vi "Main.vi"() -> ()   [LabVIEW 2020]
uses:
  Control 2.ctl
  score.ctl
  <userlib>/_NEVSTOP/Communicable State Machine(CSM)/_Support/Priority Queue/Priority Queue.lvclass/Priority Queue.ctl
  c319eba2-2b69-4508-ba06-61efdf669e7f.vi
  f21c7960-0f7f-4192-a8ac-ee65138fb98e.vi
  0e5201a1-580a-4182-a838-348a54a2e186.vi
  50275f31-ecc9-42d7-9ef1-34fd3155a618.vi
  0e7b1505-b89c-402a-9fd1-9f3cfcf1be26.vi
  d7687cdb-357b-4687-95b9-9b4cfc2d17b9.vi
  52e50a07-fba7-4300-b081-eb3bf9999503.vi
  91789a72-074d-44cf-8be7-f4eccb61965a.vi
  5ff8236f-55fa-4ae3-afc0-cb7bd4a41e4f.vi
  <userlib>/_NEVSTOP/Communicable State Machine(CSM)/_Polymophic/Build No-Reply Asynchronous Message with Arguments.vi
  939ea49c-9fb9-49f6-a0c7-57a14fefe734.vi
  03371d6b-8044-40a1-9300-825b312c4f02.vi
  d32dd9c0-23c6-42c4-b7b9-cda287316cd3.vi
  d337f771-a6ec-4da6-9b1c-67b8dc694886.vi
  9b28357d-31d9-4419-b7a1-8921e76f82ac.vi
  67dfaec1-d8c9-4a60-939d-f2d06e17c127.vi
  ca159b87-ec92-4442-a782-4ab02e472262.vi
  a8ebcde1-3a60-408d-b02a-9696afebc65b.vi
  9c19e163-6e76-42e7-8cae-1a7d439f1586.vi
  <userlib>/_NEVSTOP/Communicable State Machine(CSM)/_Support/Process/CSMP-Async Call.vi
  <userlib>/_NEVSTOP/Communicable State Machine(CSM)/_Support/GlobalEvent/GEvt-Generate Status Log.vi
  <userlib>/_NEVSTOP/Communicable State Machine(CSM)/_Support/Process/CSMP-Broadcast.vi
  <userlib>/_NEVSTOP/Communicable State Machine(CSM)/_Support/GlobalEvent/GEvt-Generate Interrupt Log.vi
  <userlib>/_NEVSTOP/Communicable State Machine(CSM)/_Support/GlobalEvent/GEvt-Generate Register Log.vi
  <userlib>/_NEVSTOP/Communicable State Machine(CSM)/_Support/Process/CSMP-Register Status.vi
  <userlib>/_NEVSTOP/Communicable State Machine(CSM)/_Support/GlobalEvent/GEvt-Generate Unregister Log.vi
  <userlib>/_NEVSTOP/Communicable State Machine(CSM)/_Support/Process/CSMP-Unregister Status.vi
  <userlib>/_NEVSTOP/Communicable State Machine(CSM)/_Support/Process/CSMP-Sync Call.vi
  <userlib>/_NEVSTOP/Communicable State Machine(CSM)/_Support/CSMQ/_CSMObj-Unlock.vi
  <userlib>/_NEVSTOP/Communicable State Machine(CSM)/_Support/Process/CSMP-PostPostMsg.vi
  <userlib>/_NEVSTOP/Communicable State Machine(CSM)/_Support/Process/CSMP-PostSendMsg.vi
  <userlib>/_NEVSTOP/Communicable State Machine(CSM)/_Support/CSMQ/_CSMObj-Lock State.vi
  <userlib>/_NEVSTOP/Communicable State Machine(CSM)/_Support/Common/Splite Reason String Part.vi
  <userlib>/_NEVSTOP/Communicable State Machine(CSM)/_Support/Common/Trim Single line Text.vi
  <userlib>/_NEVSTOP/Communicable State Machine(CSM)/_Support/CSMQ/_CSMOFGV Release.vi
  <userlib>/_NEVSTOP/Communicable State Machine(CSM)/_Support/Common/Remove Comments from Line.vi
  <userlib>/_NEVSTOP/Communicable State Machine(CSM)/_Support/Common/Splite Single-line Message.vi
  <userlib>/_NEVSTOP/Communicable State Machine(CSM)/_Support/Common/Parse Next Single-line State.vi
  <userlib>/_NEVSTOP/Communicable State Machine(CSM)/_Support/CSMQ/_CSMOFGV Dequeue.vi
  <userlib>/_NEVSTOP/Communicable State Machine(CSM)/_Support/CSMQ/_CSMObj-Log Error if in a Remote Session.vi
  <userlib>/_NEVSTOP/Communicable State Machine(CSM)/_Support/GlobalEvent/GEvt-Generate State Change Log.vi
  <userlib>/_NEVSTOP/Communicable State Machine(CSM)/_Support/GlobalEvent/GEvt-Generate Remaining States Log.vi
  <userlib>/_NEVSTOP/Communicable State Machine(CSM)/_Support/GlobalEvent/GEvt-Generate Module Destroyed Log.vi
  <userlib>/_NEVSTOP/Communicable State Machine(CSM)/_Support/GlobalEvent/GEvt-Generate Complete Log.vi
  <userlib>/_NEVSTOP/Communicable State Machine(CSM)/_Support/GlobalEvent/GEvt-Generate Module Created Log.vi
  <userlib>/_NEVSTOP/Communicable State Machine(CSM)/_Support/GlobalEvent/Cache-GEvt Filter Object.vi
  <userlib>/_NEVSTOP/Communicable State Machine(CSM)/_Support/Common/Format Timestamp.vi
  <userlib>/_NEVSTOP/Communicable State Machine(CSM)/AdvanceAPI/CSM - Wait for Module to Be Alive.vi
  <userlib>/_NEVSTOP/Communicable State Machine(CSM)/AdvanceAPI/CSM - Send Message and Wait for Reply.vi
  <userlib>/_NEVSTOP/Communicable State Machine(CSM)/AdvanceAPI/CSM - Break Down Multiple States String.vi
  <userlib>/_NEVSTOP/Communicable State Machine(CSM)/AdvanceAPI/CSM - Compact Multiple States.vi
  <userlib>/_NEVSTOP/Communicable State Machine(CSM)/Utility/uuid.vi
  <userlib>/_NEVSTOP/Communicable State Machine(CSM)/Utility/Build Error Cluster.vi
  <userlib>/_NEVSTOP/Communicable State Machine(CSM)/Utility/Trim Both Whitespace.vi
  <userlib>/_NEVSTOP/Communicable State Machine(CSM)/AdvanceAPI/CSM - Revert Arguments-Safe String.vi
  <userlib>/_NEVSTOP/Communicable State Machine(CSM)/AdvanceAPI/CSM - Make String Arguments Safe.vi
  <userlib>/_NEVSTOP/Communicable State Machine(CSM)/_Support/CSMQ/_CSMObj-Message Check.vi
  <userlib>/_NEVSTOP/Communicable State Machine(CSM)/_Support/CSMQ/_CSMObj-Enqueue Cross-Module Message.vi
  <userlib>/_NEVSTOP/Communicable State Machine(CSM)/_Support/CSMQ/_CSMOFGV Get.vi
  <userlib>/_NEVSTOP/Communicable State Machine(CSM)/_Support/GlobalEvent/GEvt-Generate with Rule Check.vi
  <userlib>/_NEVSTOP/Communicable State Machine(CSM)/_Support/FGV-BroadcastRegistry/Cache-Broadcast Registry Search Result.vi
  <userlib>/_NEVSTOP/Communicable State Machine(CSM)/AdvanceAPI/CSM - Register Status Change.vi
  <userlib>/_NEVSTOP/Communicable State Machine(CSM)/AdvanceAPI/CSM - Unregister Status Change.vi
  <userlib>/_NEVSTOP/Communicable State Machine(CSM)/_Support/Common/Hex Str to U8 Data.vi
  <userlib>/_NEVSTOP/Communicable State Machine(CSM)/_Support/Common/Concatenate State with Arguments.vi
  <userlib>/_NEVSTOP/Communicable State Machine(CSM)/_Support/Common/U8 Data to Hex Str.vi
  <userlib>/_NEVSTOP/Communicable State Machine(CSM)/_Support/Priority Queue/Dequeue Element.vi
  <userlib>/_NEVSTOP/Communicable State Machine(CSM)/AdvanceAPI/CSM - Check If Module Exists.vi
  <userlib>/_NEVSTOP/Communicable State Machine(CSM)/AdvanceAPI/CSM - Keywords.vi
  <userlib>/_NEVSTOP/Communicable State Machine(CSM)/_Support/Priority Queue/Enqueue Element.vi
  <userlib>/_NEVSTOP/Communicable State Machine(CSM)/_Support/GlobalEvent/LogFilter/Filter Check.vi
  <userlib>/_NEVSTOP/Communicable State Machine(CSM)/_Support/CSMQ/_Obtain CSM Data Queue.vi
  <userlib>/_NEVSTOP/Communicable State Machine(CSM)/_Support/Priority Queue/Release Priority Queue.vi
  <userlib>/_NEVSTOP/Communicable State Machine(CSM)/_Support/Priority Queue/Obtain Priority Queue.vi
  <userlib>/_NEVSTOP/Communicable State Machine(CSM)/_Support/GlobalEvent/FGV-GlobalEventRef.vi
  <userlib>/_NEVSTOP/Communicable State Machine(CSM)/_Support/GlobalEvent/global-GEvnt Filter Change Flag.vi
  <userlib>/_NEVSTOP/Communicable State Machine(CSM)/FGV-GEvt Filter Obj.vi
  <userlib>/_NEVSTOP/Communicable State Machine(CSM)/_Support/CSMQ/_CSMOFGV Obtain.vi
  <userlib>/_NEVSTOP/Communicable State Machine(CSM)/_Support/GlobalEvent/LogFilter/CheckVIs/Group Check - CSM.vi
  <userlib>/_NEVSTOP/Communicable State Machine(CSM)/_Support/GlobalEvent/LogFilter/CheckVIs/Group Check - LogType.vi
  <userlib>/_NEVSTOP/Communicable State Machine(CSM)/_Support/GlobalEvent/LogFilter/CheckVIs/Group Check - State.vi
  <userlib>/_NEVSTOP/Communicable State Machine(CSM)/_Support/GlobalEvent/LogFilter/CheckVIs/CSM Check - LogType.vi
  <userlib>/_NEVSTOP/Communicable State Machine(CSM)/_Support/GlobalEvent/LogFilter/CheckVIs/CSM Check - State.vi
  <userlib>/_NEVSTOP/Communicable State Machine(CSM)/_Support/GlobalEvent/LogFilter/CheckVIs/CSM Check - StateType.vi
  <userlib>/_NEVSTOP/Communicable State Machine(CSM)/_Support/GlobalEvent/LogFilter/CheckVIs/Group Check - StateType.vi
  <userlib>/_NEVSTOP/Communicable State Machine(CSM)/_Support/CSMQ/_CSMOFGV.vi
  <userlib>/_NEVSTOP/Communicable State Machine(CSM)/_Support/Error/CSM Not Allowed Message.vi
  <userlib>/_NEVSTOP/Communicable State Machine(CSM)/_Support/GlobalEvent/FGV-StatusChangeEventRef.vi
  <userlib>/_NEVSTOP/Communicable State Machine(CSM)/_Support/FGV-BroadcastRegistry/global-CSMQ FGV Change Flag.vi
  <userlib>/_NEVSTOP/Communicable State Machine(CSM)/_Support/FGV-BroadcastRegistry/global-Broadcast Cache Change Flag.vi
  <userlib>/_NEVSTOP/Communicable State Machine(CSM)/_Support/BroadcastRegistry/HelperVI/Broadcast Item Key.vi
  <userlib>/_NEVSTOP/Communicable State Machine(CSM)/_Support/FGV-BroadcastRegistry/FGV-BroadcastRegistry.vi
  <userlib>/_NEVSTOP/Communicable State Machine(CSM)/_Support/Message/Parse Register Message.vi
  <userlib>/_NEVSTOP/Communicable State Machine(CSM)/_Support/Message/Parse Unregister Message.vi
  <userlib>/_NEVSTOP/Communicable State Machine(CSM)/addons/API-String-Arugments-Support/_Support/Data To API String Arguments.vi
  <userlib>/_NEVSTOP/Communicable State Machine(CSM)/_Support/Error/CSM No Target Error.vi
  <userlib>/_NEVSTOP/Communicable State Machine(CSM)/addons/API-String-Arugments-Support/_Support/Convert API String Arguments to Data(variant).vi
  <userlib>/_NEVSTOP/Communicable State Machine(CSM)/_Support/Message/Parse State with Arguments String.vi
  <userlib>/_NEVSTOP/Communicable State Machine(CSM)/_Support/Priority Queue/Priority Queue.lvclass
  <userlib>/_NEVSTOP/Communicable State Machine(CSM)/Communicable State Machine.lvlib
panel:
  out "time":dbl
  in  "Stop":bool
  out "State History":string="\r"
  in  "Name(\"\" to use uuid)":string="Main"
  in  "Init State(\"Macro: Initialize\")":string="Macro: Initialize"
  in  "Tab Control":T1
  in  "exit":bool
  in  "register":bool
  in  "log":bool
  in  "username":string
  in  "password":string
  in  "level":enum16{"simple", "medium", "hard"}(ring)
  in  "newgame":bool
  in  "logout":bool
  in  "ranking":bool
  in  "continue":bool
  in  "Boolean 4":bool
  in  "Boolean 3":bool
  in  "Boolean 2":bool
  in  "Boolean1":bool
  in  "exit2":bool
  in  "start2":bool
  in  "save":bool
  in  "pause":bool
  out "Score":T2
  out "Countdown":dbl
  in  "update":bool
  in  "Top":i32=1 min=1 max=10 step=1
  out "Data":string[][](array[string])
  in  "exit3":bool
  # "Player"
  # "Score"
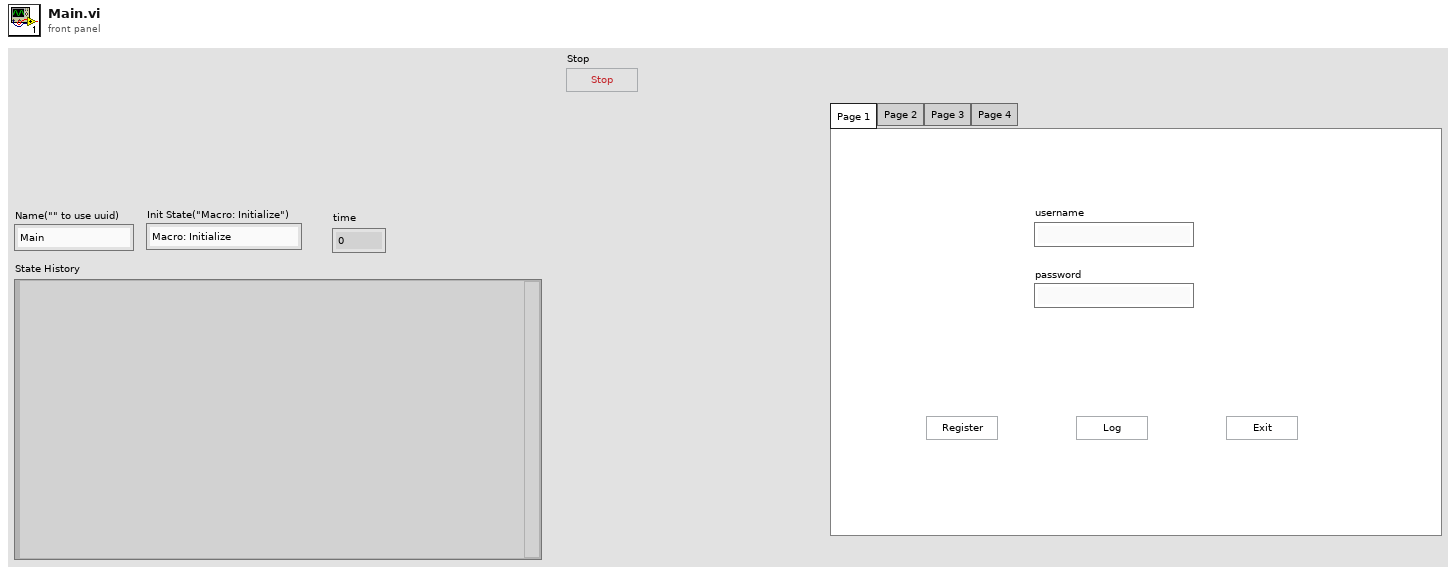
[diagram p1: front panel]
types:
  T1 = typedef "Control 2.ctl" = enum32{"Page 1", "Page 2", "Page 3", "Page 4"}
  T2 = typedef "score.ctl" = i32
  T3 = enum8{"Enabled", "Disabled", "Disabled and Grayed Out"}
  T4 = enum32{"Invalid", "Standard", "Closed", "Hidden", "Minimized", "Maximized"}
  T5 = enum32{"invalid app kind", "Development System", "Run Time System", "Student Edition", "Embedded LabVIEW", "Evaluation", "Custom"}
  T6 = typedef "Communicable State Machine.lvlib/_CSM_Response Source Message.ctl" = cluster{"‘State":string, "’Arguments":string, "’Error":errorcluster}
  T7 = cluster{"Tab Control":refnum<vi>, "start2":refnum<vi>, "Boolean1":refnum<vi>, "Boolean 3":refnum<vi>, "Boolean 4":refnum<vi>, "Boolean 2":refnum<vi>, "Core":cluster{"Current VI Reference":refnum<vi>, "Close Panel on Exit?":bool}, "rank":string[][], "ID":cluster{"username":string, "password":string}, "score":i32, "timeseq":cluster{"time":i32, "SEQ":i32[]}, "appended path":path, "start time":dbl, "Countdown":refnum<vi>}
  T8 = cluster{"Current VI Reference":refnum<vi>, "Close Panel on Exit?":bool}
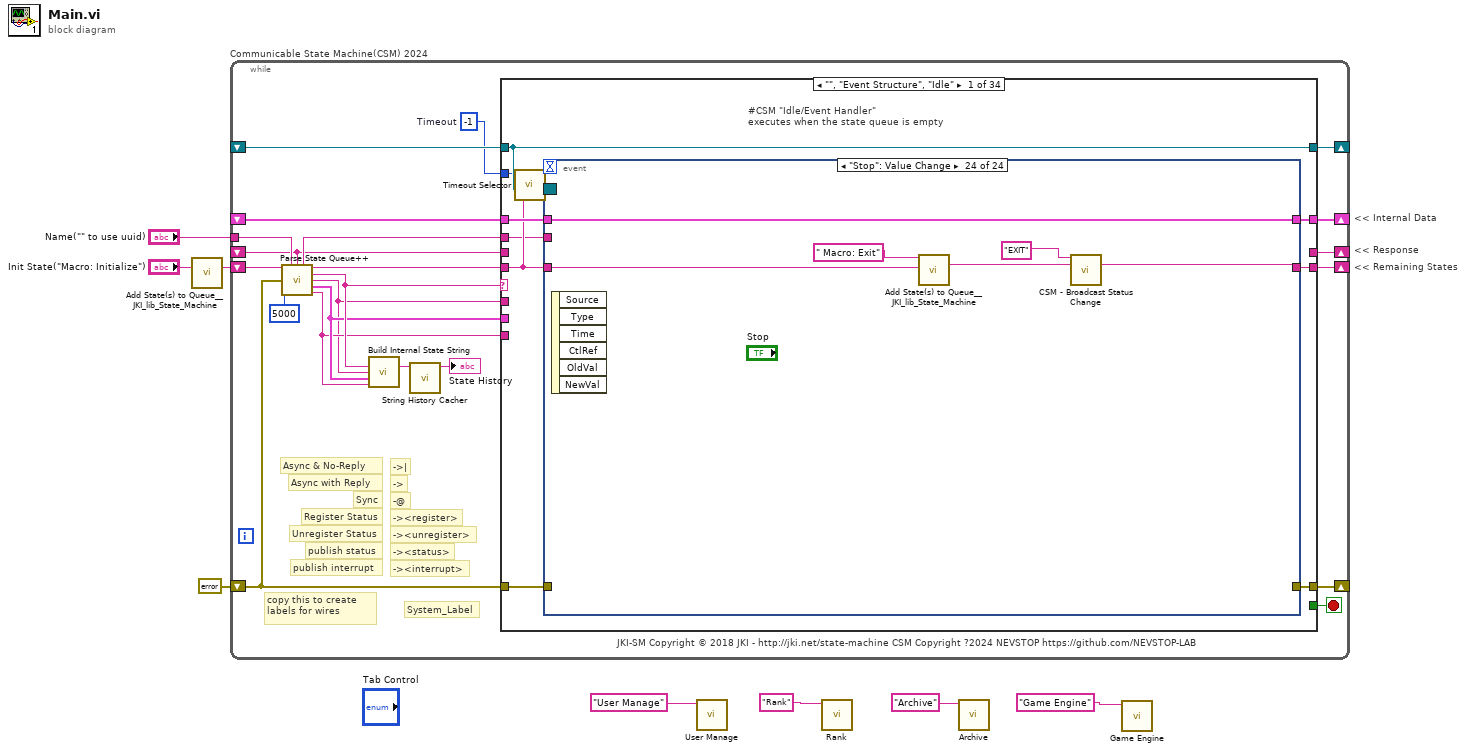
[diagram p0: block diagram]
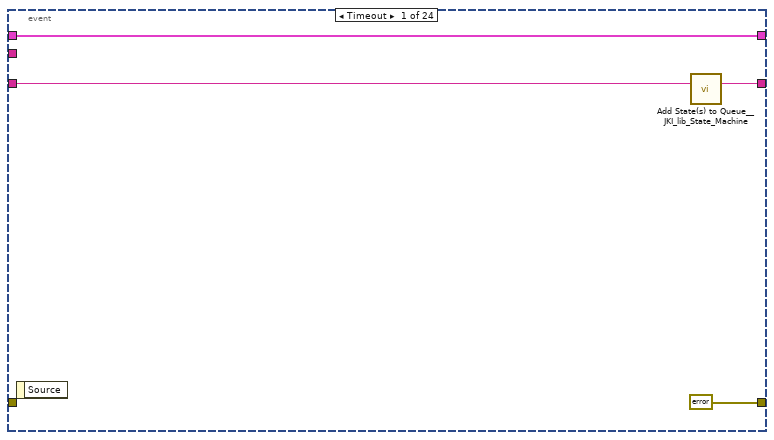
[diagram p2: hidden frame]
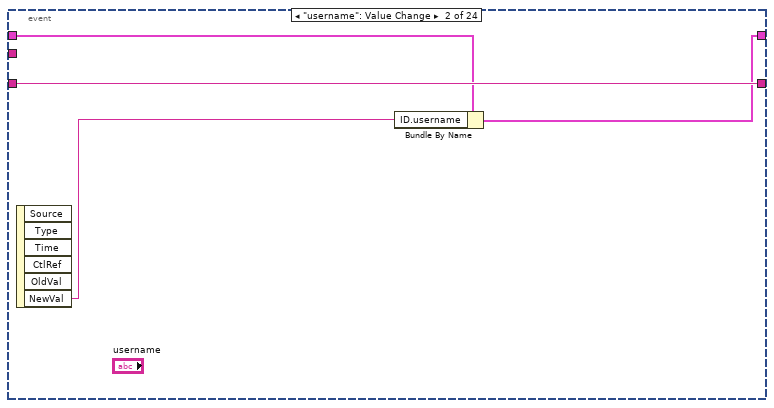
[diagram p3: hidden frame]
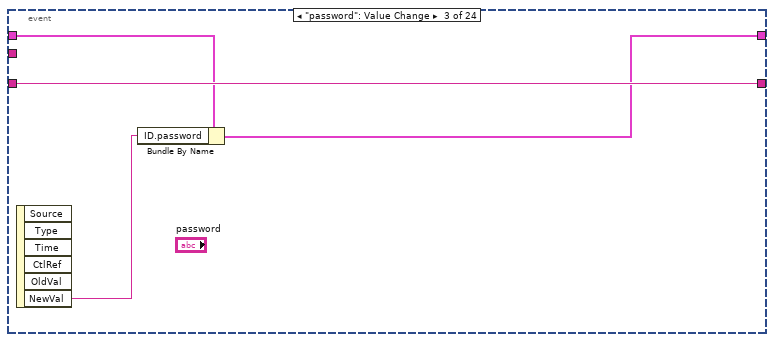
[diagram p4: hidden frame]
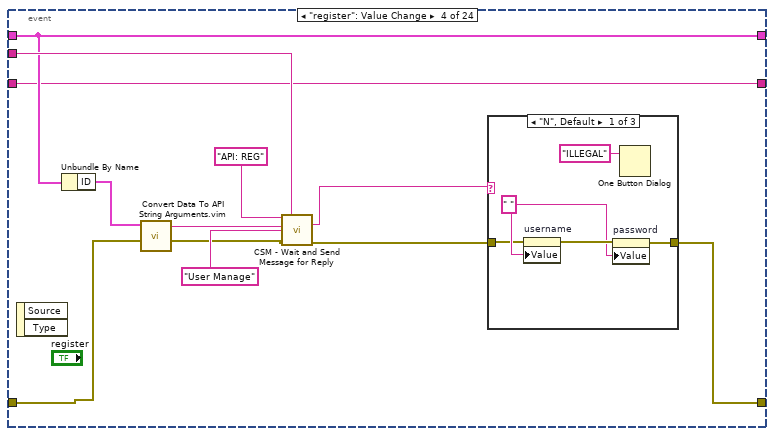
[diagram p5: hidden frame]
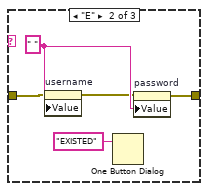
[diagram p6: hidden frame]
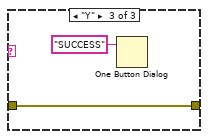
[diagram p7: hidden frame]
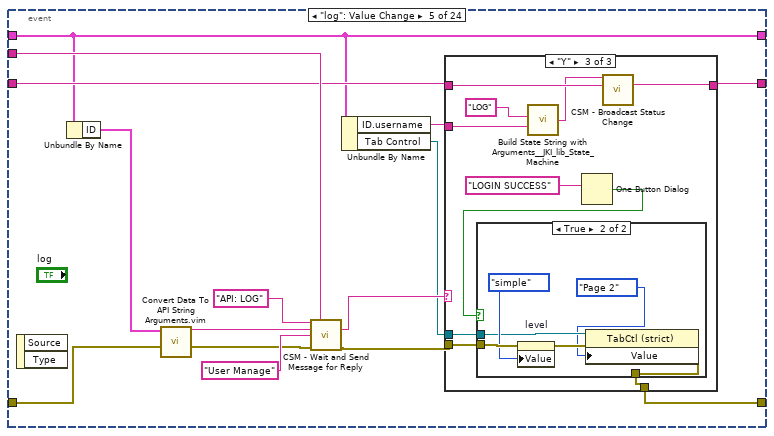
[diagram p8: hidden frame]
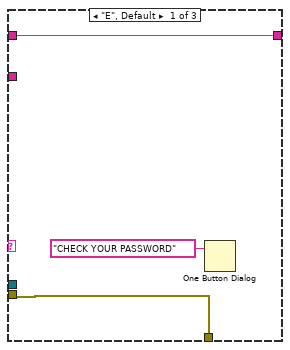
[diagram p9: hidden frame]
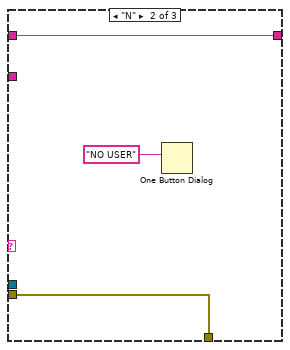
[diagram p10: hidden frame]
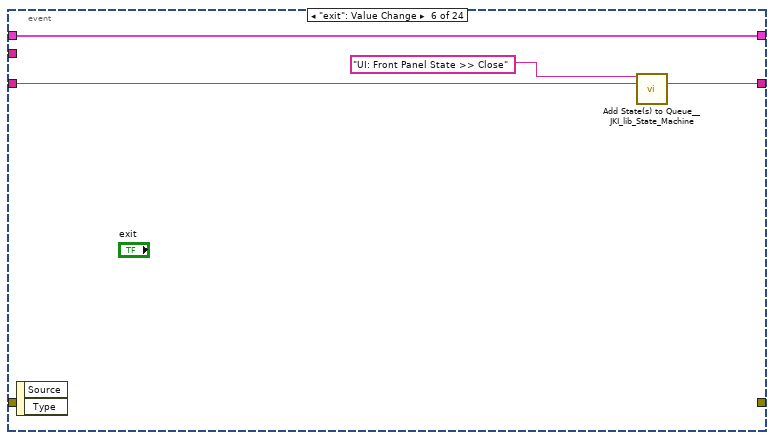
[diagram p12: hidden frame]
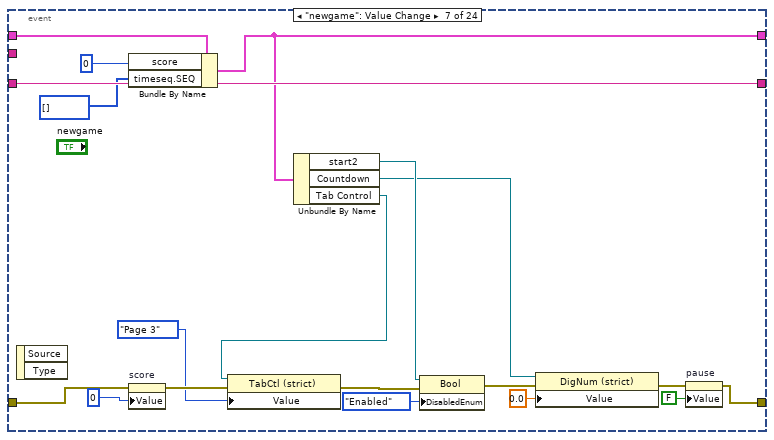
[diagram p13: hidden frame]
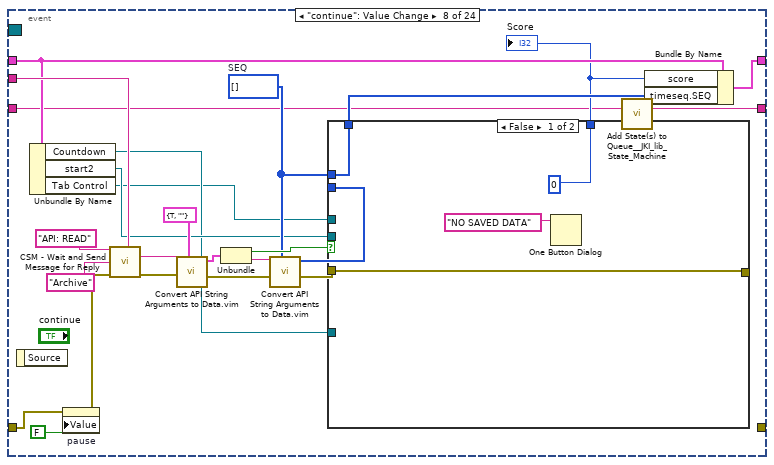
[diagram p14: hidden frame]
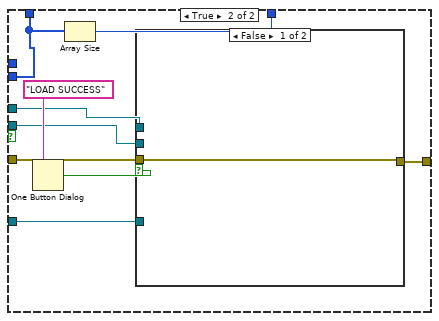
[diagram p15: hidden frame]
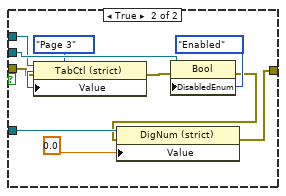
[diagram p16: hidden frame]
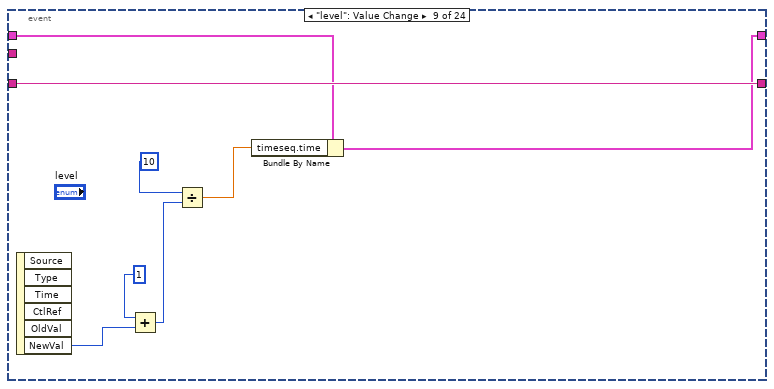
[diagram p17: hidden frame]
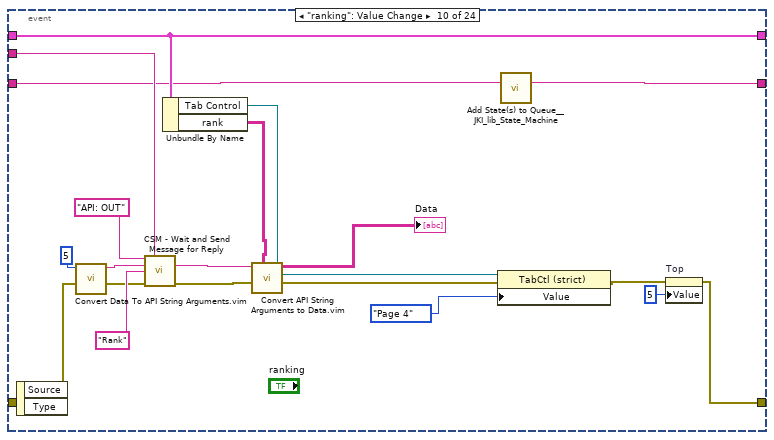
[diagram p18: hidden frame]
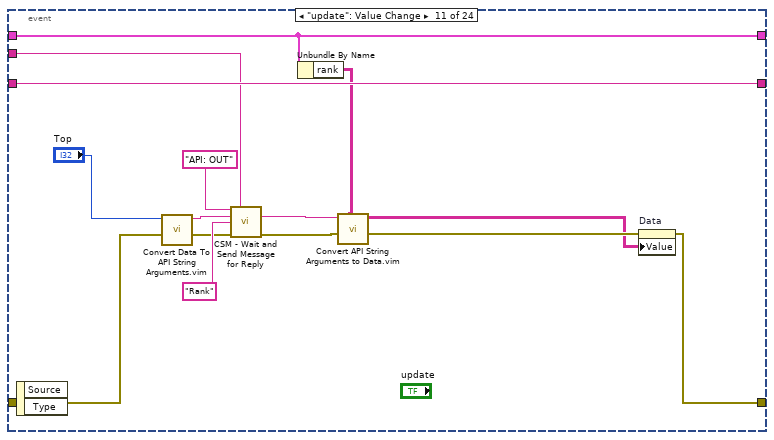
[diagram p19: hidden frame]
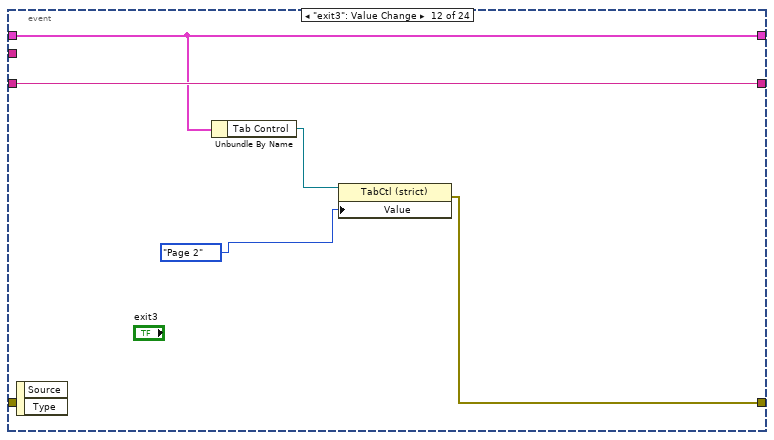
[diagram p20: hidden frame]
diagram:
  # "<< Internal Data"
  # "<< Response"
  # "<< Remaining States"
  n1 = call <vilib>:"Add State(s) to Queue__JKI_lib_State_Machine.vi"("State(s) in (\"\")"="Init State(\"Macro: Initialize\")") -> ("States Out"=w5:string)  [unwired: 14 in]
  n2 = while "Communicable State Machine(CSM) 2024" {
    shift-right: [w25] -> _
    shift-left: _ -> [w24]
    shift-right: [w28] -> _
    shift-left: errorcluster {"status"=FALSE, "code"=0, "source"=""} ("error out") -> [w23]
    shift-right: [w27] -> _
    shift-left: w5 -> [w29]
    tunnel: "Name(\"\" to use uuid)" -> [w18]
    shift-right: [w21] -> _
    shift-left: _ -> [w11]
    shift-right: [w20] -> _
    shift-left: _ -> [w19]
    stop <- w26 stop-if-true
    w9 = -1  # Timeout
    # "-><interrupt>"
    # "-><status>"
    # "-><unregister>"
    # "-><register>"
    # "-@"
    # "->"
    # "->|"
    # "publish interrupt"
    # "publish status"
    # "Unregister Status"
    # "Register Status"
    # "Sync"
    # "Async with Reply"
    # "Async & No-Reply"
    # "copy this to create labels for wires"
    # "System_Label"
    # "JKI-SM Copyright © 2018 JKI - http://jki.net/state-machine CSM Copyright ?2024 NEVSTOP https://github.com/NEVSTOP-LAB"
    n3 = call <userlib>:"Parse State Queue++.vi"("State Queue"=w29, "Name(\"\" to use uuid)"=w18, "Response Arguments"=w11, "Error In (no error)"=w23, "Response Timeout(5000ms)"=5000 ("Response Timeout(1000ms)")) -> ("Name Used"=w12:string, "Remaining States"=w30:string, "Current State"=w15:string, "Arguments"=w10:string, ">> Response Source Message >>"=w14:T6, ">> Source CSM >>"=w13:string)  [unwired: 5 in]
    n4 = call <userlib>:"Build Internal State String.vi"("State"=w15, "Arguments (\"\")"=w10, ">> Response Source Message >>"=w14, "Source (\"\")"=w13) -> ("State with Arguments"=w16:string)  [unwired: 11 in]
    n5 = call <userlib>:"String History Cacher.vi"("String"=w16) -> ("String Cache"=→"State History":string)  [unwired: 10 in]
    n6 = case shown="\"\", \"Event Structure\", \"Idle\"" w15 {
      selector: w15 -> [_ _ _ w405 _ _ _ _ _ _ _ _ _ _ _ _ _ _ _ _ _ _ _ _ _ _ _ _ _ _ _ _ _ _]
      tunnel: w30 -> [w34 w397 w402 w411 w417 w424 w451 w459 w466 w476 w485 w498 w503 w507 w527 w533 w537 w544 w548 w552 w577 w583 w596 w660 w665 w676 w679 w688 w731 w750 w770 w786 w801 w821]
      tunnel: w10 -> [_ _ _ _ _ w422 w447 w454 w462 w470 _ _ _ _ _ _ _ _ _ _ _ w579 w593 _ _ _ _ w692 w728 _ _ _ _ _]
      tunnel: w24 -> [w39 w396 w399 w409 w416 w430 w452 w457 w464 w474 w484 w492 w501 w505 _ w529 w535 w543 w547 w550 w574 w581 w594 w658 w663 w674 w678 w691 w724 w734 w777 w784 w798 w810]
      tunnel: [w38 _ w400 w403 w418 errorcluster {"status"=FALSE, "code"=0, "source"=""} ("error out") w444 w453 w460 w473 _ _ _ _ _ w530 _ w538 w546 _ w554 w580 w589 _ _ _ _ w684 w726 w739 w756 _ w794 w815] -> w28
      tunnel: w23 -> [w32 _ w400 w404 w418 w428 w445 w455 w461 _ _ _ _ _ _ _ _ _ _ _ w557 _ _ _ _ _ _ _ w727 w737 w762 _ w788 w802]
      tunnel: [w40 w397 w401 w410 w417 w426 w450 w458 w465 w477 w485 w497 w502 w506 w526 w532 w536 w544 w548 w551 w576 w582 w595 w659 w664 w675 w679 w689 w730 w751 w771 w785 w800 w820] -> w27
      tunnel: [_ _ _ _ _ _ TRUE _ _ _ _ _ TRUE _ _ _ _ _ _ _ _ _ _ _ _ _ _ _ _ _ _ _ _ _] -> w26
      tunnel: [w37 w396 w399 w409 w416 w430 w452 w457 w464 w475 w484 w496 w501 w505 w525 w529 w535 w543 w547 w550 w574 w581 w594 w658 w663 w674 w678 w686 w724 w733 w781 w784 w798 w810] -> w25
      tunnel: w13 -> [_ _ _ _ _ w421 _ _ _ w471 _ _ _ _ _ _ _ _ _ _ _ _ _ _ _ _ _ _ _ _ _ _ _ _]
      tunnel: w14 -> [_ _ _ _ _ w420 _ _ _ w472 _ _ _ _ _ _ _ _ _ _ _ _ _ _ _ _ _ _ _ _ _ _ _ _]
      tunnel: [_ _ _ "" w412 w419 _ _ _ _ _ _ _ _ _ _ _ _ _ _ _ _ _ _ _ _ _ _ _ _ _ _ _ _] -> w21
      tunnel: [w36 w395 w398 w407 w415 w429 w448 w456 w463 w478 w483 w486 w499 w504 w523 w528 w534 w542 w545 w549 w575 w578 w592 w657 w661 w667 w677 w694 w729 w752 w782 w783 w799 w819] -> w20
      tunnel: w19 -> [w36 w395 w398 w407 w415 w429 w448 w456 w463 w478 w483 w486 w499 w504 w523 w528 w534 _ w545 w549 w575 w578 w592 w657 w661 w667 w677 w694 w729 w752 w782 w783 w799 w819]
      tunnel: w12 -> [w33 _ _ w406 _ _ w446 _ _ _ _ _ _ _ _ _ _ w541 _ _ _ _ _ _ _ _ _ _ _ _ _ _ _ _]
      tunnel: w11 -> [_ _ _ _ _ w419 _ _ _ _ _ _ _ _ _ _ _ _ _ _ _ _ _ _ _ _ _ _ _ _ _ _ _ _]
      tunnel: w9 -> [w31 _ _ _ _ _ _ _ _ _ _ _ _ _ _ _ _ _ _ _ _ _ _ _ _ _ _ _ _ _ _ _ _ _]
      frame "", "Event Structure", "Idle" {
        # "#CSM \"Idle/Event Handler\"\nexecutes when the state queue is empty"
        n7 = call <userlib>:"Timeout Selector.vi"("Remaining States"=w34, "Timeout Expected"=w31) -> ("Timeout"=w35:i32)  [unwired: 5 in]
        n8 = event shown="[23] \"Stop\": Value Change" {
          selector: w36 -> [_ _ _ _ _ _ _ _ _ _ _ _ _ _ _ _ _ _ _ _ _ _ _ _]
          dyn-events: _ -> [_ _ _ _ _ _ _ _ _ _ _ _ _ _ _ _ _ _ _ _ _ _ _ _]
          timeout: w35 -> [_ _ _ _ _ _ _ _ _ _ _ _ _ _ _ _ _ _ _ _ _ _ _ _]
          tunnel: w34 -> [w44 w48 w52 w56 w82 w115 w137 w138 w194 w195 w229 w234 w246 w254 w266 w283 w329 w335 w347 w360 w373 w382 w388 w390]
          tunnel: [w43 w48 w52 w56 w83 w117 w137 w139 w194 w196 w229 w234 w246 w260 w267 w284 w328 w336 w348 w361 w374 w382 w387 w392] -> w40
          tunnel: w39 -> [w42 w47 w50 w62 w81 w118 w136 w159 w193 w205 w219 w233 w240 w259 w268 w291 w325 w333 w344 w358 w371 w383 w386 w394]
          tunnel: [errorcluster {"status"=FALSE, "code"=0, "source"=""} ("error out") _ _ w53 w84 _ w121 _ _ w202 w216 w230 w244 w249 w262 w280 w320 w331 w345 w356 w369 _ _ _] -> w38
          tunnel: [w42 w46 w49 w62 w81 w118 w132 w158 w188 w205 w219 w233 w241 w259 w268 w291 w325 w333 w344 w358 w371 w383 w386 w394] -> w37
          tunnel: w33 -> [_ _ _ w64 w85 _ _ w162 _ w213 w221 _ _ _ _ w281 _ _ _ _ _ _ _ _]
          tunnel: w32 -> [_ _ _ w58 w86 _ w135 w144 _ w207 w222 _ w237 w261 w263 w290 w322 _ _ _ _ _ _ _]
          event Timeout {
            n9 = event-data() -> ()  [unwired: 1 in, 1 out]
            n10 = call <vilib>:"Add State(s) to Queue__JKI_lib_State_Machine.vi"("State(s) in (\"\")"=w44) -> ("States Out"=w43:string)  [unwired: 14 in]
          }
          event "username": Value Change {
            n11 = event-data() -> ("NewVal"=w45:string)  [unwired: 1 in, 5 out]
            n12 = Bundle By Name(cluster=w47, "ID.username"=w45) -> (w46:T7)
          }
          event "password": Value Change {
            n13 = event-data() -> ("NewVal"=w51:string)  [unwired: 1 in, 5 out]
            n14 = Bundle By Name(cluster=w50, "ID.password"=w51) -> (w49:T7)
          }
          event "register": Value Change {
            n15 = event-data() -> ()  [unwired: 1 in, 2 out]
            n16 = Unbundle By Name(w62) -> ("ID"=w61:cluster{"username":string, "password":string})
            n17 = call "Convert Data To API String Arguments.vim"("error in (no error)"=w58, "data"=w61) -> ("error out"=w57:errorcluster, "String"=w60:string)  [unwired: 6 in]
            n18 = call <userlib>:"CSM - Wait and Send Message for Reply.vi"("State"="API: REG", "Current Module(\"\" to generate a ID)"=w64, "Arguments (\"\")"=w60, "Target Module"="User Manage", "Error In (no error)"=w57) -> ("Response"=w55:string, "error out"=w54:errorcluster)  [unwired: 8 in, 1 out]
            n19 = case shown="\"N\", Default" w55 {
              tunnel: w54 -> [w65 w72 w75]
              tunnel: [w66 w70 w75] -> w53
              frame "N", Default {
                w67 = " " ("username")
                n20 = property on="username" class="Str"(error in=w65, "Value"=w67) -> (error out=w68:errorcluster)  [unwired: 1 in, 1 out]
                n21 = property on="password" class="Str"(error in=w68, "Value"=w67) -> (error out=w66:errorcluster)  [unwired: 1 in, 1 out]
                n22 = One Button Dialog(message="ILLEGAL") -> ()  [unwired: 1 in, 1 out]
              }
              frame "E" {
                w73 = " " ("username")
                n23 = property on="username" class="Str"(error in=w72, "Value"=w73) -> (error out=w71:errorcluster)  [unwired: 1 in, 1 out]
                n24 = One Button Dialog(message="EXISTED") -> ()  [unwired: 1 in, 1 out]
                n25 = property on="password" class="Str"(error in=w71, "Value"=w73) -> (error out=w70:errorcluster)  [unwired: 1 in, 1 out]
              }
              frame "Y" {
                n26 = One Button Dialog(message="SUCCESS") -> ()  [unwired: 1 in, 1 out]
              }
            }
          }
          event "log": Value Change {
            n27 = event-data() -> ()  [unwired: 1 in, 2 out]
            n28 = Unbundle By Name(w81) -> ("ID"=w90:cluster{"username":string, "password":string})
            n29 = call "Convert Data To API String Arguments.vim"("error in (no error)"=w86, "data"=w90) -> ("error out"=w87:errorcluster, "String"=w89:string)  [unwired: 6 in]
            n30 = call <userlib>:"CSM - Wait and Send Message for Reply.vi"("State"="API: LOG", "Current Module(\"\" to generate a ID)"=w85, "Arguments (\"\")"=w89, "Target Module"="User Manage", "Error In (no error)"=w87) -> ("Response"=w78:string, "error out"=w79:errorcluster)  [unwired: 8 in, 1 out]
            n31 = Unbundle By Name(w81) -> ("ID.username"=w80:string, "Tab Control"=w77:refnum<vi>)
            n32 = case shown="\"Y\"" w78 {
              tunnel: w79 -> [w93 w96 w105]
              tunnel: [w93 w96 w104] -> w84
              tunnel: [w92 w95 w102] -> w83
              tunnel: w82 -> [w92 w95 w103]
              tunnel: w80 -> [_ _ w100]
              tunnel: w77 -> [_ _ w98]
              frame "E", Default {
                n33 = One Button Dialog(message="CHECK YOUR PASSWORD") -> ()  [unwired: 1 in, 1 out]
              }
              frame "N" {
                n34 = One Button Dialog(message="NO USER") -> ()  [unwired: 1 in, 1 out]
              }
              frame "Y" {
                n35 = call <vilib>:"Build State String with Arguments__JKI_lib_State_Machine.vi"("Arguments (\"\")"=w100, "State"="LOG") -> ("State with Arguments"=w101:string)  [unwired: 4 in]
                n36 = One Button Dialog(message="LOGIN SUCCESS") -> (true=w106:bool)  [unwired: 1 in]
                n37 = case shown="True" w106 {
                  tunnel: w105 -> [w108 w114]
                  tunnel: [w108 w110] -> w104
                  tunnel: w98 -> [_ w111]
                  frame False {
                  }
                  frame True {
                    n38 = property on="level" class="Enum (strict)"(error in=w114, "Value"=enum16{"simple", "medium", "hard"}."simple" ("level")) -> (error out=w112:errorcluster)  [unwired: 1 in, 1 out]
                    n39 = property class="TabCtl (strict)"(reference=w111, error in=w112, "Value"=Control_2."Page 2" ("Tab Control")) -> (error out=w110:errorcluster)  [unwired: 1 out]
                  }
                }
                n40 = call <userlib>:"CSM - Broadcast Status Change.vi"("Status with Arguments"=w101, "State Queue"=w103) -> ("Remaining States"=w102:string)  [unwired: 13 in]
              }
            }
          }
          event "exit": Value Change {
            n41 = event-data() -> ()  [unwired: 1 in, 2 out]
            n42 = call <vilib>:"Add State(s) to Queue__JKI_lib_State_Machine.vi"("State(s) in Front (\"\")"="UI: Front Panel State >> Close" ("State(s) in Front (\"\")"), "State(s) in (\"\")"=w115) -> ("States Out"=w117:string)  [unwired: 13 in]
          }
          event "newgame": Value Change {
            n43 = event-data() -> ()  [unwired: 1 in, 2 out]
            n44 = Bundle By Name(cluster=w136, "score"=0, "timeseq.SEQ"=i32[] [] ("SEQ")) -> (w132:T7)
            n45 = property on="score" class="DigNum (strict)"(error in=w135, "Value"=T2 0 ("score")) -> (error out=w126:errorcluster)  [unwired: 1 in, 1 out]
            n46 = Unbundle By Name(w132) -> ("start2"=w131:refnum<vi>, "Countdown"=w129:refnum<vi>, "Tab Control"=w123:refnum<vi>)
            n47 = property class="TabCtl (strict)"(reference=w123, error in=w126, "Value"=Control_2."Page 3" ("Tab Control")) -> (error out=w125:errorcluster)  [unwired: 1 out]
            n48 = property class="Bool"(reference=w131, error in=w125, "DisabledEnum"=T3."Enabled" ("Disabled")) -> (error out=w128:errorcluster)  [unwired: 1 out]
            n49 = property class="DigNum (strict)"(reference=w129, error in=w128, "Value"=0.0) -> (error out=w122:errorcluster)  [unwired: 1 out]
            n50 = property on="pause" class="Bool (strict)"(error in=w122, "Value"=FALSE ("pause")) -> (error out=w121:errorcluster)  [unwired: 1 in, 1 out]
          }
          event "continue": Value Change {
            w147 = i32[] []  # SEQ
            n51 = event-data() -> ()  [unwired: 1 in, 1 out]
            n52 = Unbundle By Name(w159) -> ("Countdown"=w141:refnum<vi>, "start2"=w142:refnum<vi>, "Tab Control"=w140:refnum<vi>)
            n53 = property on="pause" class="Bool (strict)"(error in=w144, "Value"=FALSE ("pause")) -> (error out=w143:errorcluster)  [unwired: 1 in, 1 out]
            n54 = call <userlib>:"CSM - Wait and Send Message for Reply.vi"("State"="API: READ", "Current Module(\"\" to generate a ID)"=w162, "Target Module"="Archive", "Error In (no error)"=w143) -> ("Response"=w156:string, "error out"=w157:errorcluster)  [unwired: 9 in, 1 out]
            n55 = call "Convert API String Arguments to Data.vim"("Type"=cluster{"found?":bool, "value":string} {"found?"=TRUE, "value"=""}, "error in (no error)"=w157, "String"=w156) -> ("error"=w150:errorcluster, "Data"=w154:cluster{"found?":bool, "value":string})  [unwired: 5 in]
            n56 = Unbundle(w154) -> ("found?"=w153:bool, "value"=w152:string)
            n57 = call "Convert API String Arguments to Data.vim"("Type"=w147, "error in (no error)"=w150, "String"=w152) -> ("error"=w149:errorcluster, "Data"=w151:i32[])  [unwired: 5 in]
            n58 = case shown="False" w153 {
              tunnel: w149 -> [w164 w173]
              tunnel: [0 ("score") w171] -> w146
              tunnel: [w164 w172] -> _
              tunnel: w151 -> [_ w170]
              tunnel: [w163 w170] -> w148
              tunnel: w147 -> [w163 _]
              tunnel: w142 -> [_ w169]
              tunnel: w141 -> [_ w168]
              tunnel: w140 -> [_ w167]
              frame False {
                n59 = One Button Dialog(message="NO SAVED DATA") -> ()  [unwired: 1 in, 1 out]
              }
              frame True {
                n60 = One Button Dialog(message="LOAD SUCCESS") -> (true=w174:bool)  [unwired: 1 in]
                n61 = Array Size(array=w170) -> (size(s)=w171:i32)
                n62 = case shown="False" w174 {
                  tunnel: w173 -> [w176 w178]
                  tunnel: [w176 w181] -> w172
                  tunnel: w169 -> [_ w184]
                  tunnel: w168 -> [_ w183]
                  tunnel: w167 -> [_ w177]
                  frame False {
                  }
                  frame True {
                    n63 = property class="TabCtl (strict)"(reference=w177, error in=w178, "Value"=Control_2."Page 3" ("Tab Control")) -> (error out=w179:errorcluster)  [unwired: 1 out]
                    n64 = property class="Bool"(reference=w184, error in=w179, "DisabledEnum"=T3."Enabled" ("Disabled")) -> (error out=w182:errorcluster)  [unwired: 1 out]
                    n65 = property class="DigNum (strict)"(reference=w183, error in=w182, "Value"=0.0) -> (error out=w181:errorcluster)  [unwired: 1 out]
                  }
                }
              }
            }
            "Score" <- w146
            n66 = call <vilib>:"Add State(s) to Queue__JKI_lib_State_Machine.vi"("State(s) in (\"\")"=w138) -> ("States Out"=w139:string)  [unwired: 14 in]
            n67 = Bundle By Name(cluster=w159, "score"=w146, "timeseq.SEQ"=w148) -> (w158:T7)
          }
          event "level": Value Change {
            n68 = event-data() -> ("NewVal"=w192:enum16{"simple", "medium", "hard"})  [unwired: 1 in, 5 out]
            n69 = Add(x=1, y=w192) -> (x+y=w190:i32)
            n70 = Divide(x=10, y=w190) -> (x/y=w187:dbl)
            n71 = Bundle By Name(cluster=w193, "timeseq.time"=w187) -> (w188:T7)
          }
          event "ranking": Value Change {
            n72 = event-data() -> ()  [unwired: 1 in, 2 out]
            n73 = call "Convert Data To API String Arguments.vim"("error in (no error)"=w207, "data"=5 ("top")) -> ("error out"=w208:errorcluster, "String"=w209:string)  [unwired: 6 in]
            n74 = call <userlib>:"CSM - Wait and Send Message for Reply.vi"("State"="API: OUT", "Current Module(\"\" to generate a ID)"=w213, "Arguments (\"\")"=w209, "Target Module"="Rank", "Error In (no error)"=w208) -> ("Response"=w211:string, "error out"=w210:errorcluster)  [unwired: 8 in, 1 out]
            n75 = Unbundle By Name(w205) -> ("Tab Control"=w197:refnum<vi>, "rank"=w204:string[][])
            n76 = call "Convert API String Arguments to Data.vim"("Type"=w204, "error in (no error)"=w210, "String"=w211) -> ("error"=w200:errorcluster, "Data"=→"Data":string[][])  [unwired: 5 in]
            n77 = property class="TabCtl (strict)"(reference=w197, error in=w200, "Value"=Control_2."Page 4" ("Tab Control")) -> (error out=w199:errorcluster)  [unwired: 1 out]
            n78 = call <vilib>:"Add State(s) to Queue__JKI_lib_State_Machine.vi"("State(s) in (\"\")"=w195) -> ("States Out"=w196:string)  [unwired: 14 in]
            n79 = property on="Top" class="DigNum (strict)"(error in=w199, "Value"=5 ("top")) -> (error out=w202:errorcluster)  [unwired: 1 in, 1 out]
          }
          event "update": Value Change {
            n80 = event-data() -> ()  [unwired: 1 in, 2 out]
            n81 = call "Convert Data To API String Arguments.vim"("error in (no error)"=w222, "data"="Top") -> ("error out"=w223:errorcluster, "String"=w224:string)  [unwired: 6 in]
            n82 = call <userlib>:"CSM - Wait and Send Message for Reply.vi"("State"="API: OUT", "Current Module(\"\" to generate a ID)"=w221, "Arguments (\"\")"=w224, "Target Module"="Rank", "Error In (no error)"=w223) -> ("Response"=w226:string, "error out"=w225:errorcluster)  [unwired: 8 in, 1 out]
            n83 = Unbundle By Name(w219) -> ("rank"=w218:string[][])
            n84 = call "Convert API String Arguments to Data.vim"("Type"=w218, "error in (no error)"=w225, "String"=w226) -> ("error"=w217:errorcluster, "Data"=w215:string[][])  [unwired: 5 in]
            n85 = property on="Data" class="Arr (strict)"(error in=w217, "Value"=w215) -> (error out=w216:errorcluster)  [unwired: 1 in, 1 out]
          }
          event "exit3": Value Change {
            n86 = event-data() -> ()  [unwired: 1 in, 2 out]
            n87 = Unbundle By Name(w233) -> ("Tab Control"=w232:refnum<vi>)
            n88 = property class="TabCtl (strict)"(reference=w232, "Value"=Control_2."Page 2" ("Tab Control")) -> (error out=w230:errorcluster)  [unwired: 1 in, 1 out]
          }
          event "logout": Value Change {
            w242 = "" ("ID.username")
            w243 = "" ("password")
            n89 = event-data() -> ()  [unwired: 1 in, 2 out]
            n90 = Unbundle By Name(w240) -> ("Tab Control"=w239:refnum<vi>)
            n91 = Bundle By Name(cluster=w240, "ID.username"=w242, "ID.password"=w242, "timeseq.time"=10) -> (w241:T7)
            n92 = property class="TabCtl (strict)"(reference=w239, error in=w237, "Value"=Control_2."Page 1" ("Tab Control")) -> (error out=w236:errorcluster)  [unwired: 1 out]
            n93 = property on="password" class="Str"(error in=w236, "Value"=w243) -> (error out=w245:errorcluster)  [unwired: 1 in, 1 out]
            n94 = property on="username" class="Str"(error in=w245, "Value"=w243) -> (error out=w244:errorcluster)  [unwired: 1 in, 1 out]
          }
          event "start2": Value Change {
            n95 = event-data() -> ()  [unwired: 1 in, 4 out]
            n96 = Unbundle By Name(w259) -> ("timeseq"=w248:cluster{"time":i32, "SEQ":i32[]})
            n97 = call "Convert Data To API String Arguments.vim"("error in (no error)"=w261, "data"=w248) -> ("error out"=w250:errorcluster, "String"=w257:string)  [unwired: 6 in]
            n98 = call <vilib>:"Add State(s) to Queue__JKI_lib_State_Machine.vi"("State(s) in (\"\")"=w254) -> ("States Out"=w255:string)  [unwired: 14 in]
            n99 = call-poly <userlib>:"Build Message with Arguments++.vi"("State with Arguments"="API: SEQ" ("State"), "Arguments (\"\")"=w257, "Target Module (\"\")"="Game Engine" ("Target Module")) -> ("State with Arguments out"=w253:string)  [unwired: 12 in]
            n100 = call <vilib>:"Add State(s) to Queue__JKI_lib_State_Machine.vi"("State(s) in Front (\"\")"="Action: DISABLE" ("State(s) in Front (\"\")"), "State(s) in (\"\")"=w253) -> ("States Out"=w247:string)  [unwired: 13 in]
            n101 = property on="start2" class="Bool"(error in=w250, "DisabledEnum"=T3."Disabled and Grayed Out" ("Disabled")) -> (error out=w249:errorcluster)  [unwired: 1 in, 1 out]
            n102 = call <vilib>:"Add State(s) to Queue__JKI_lib_State_Machine.vi"("State(s) in Front (\"\")"=w247, "State(s) in (\"\")"=w255) -> ("States Out"=w260:string)  [unwired: 13 in]
          }
          event "pause": Value Change {
            n103 = event-data() -> ("NewVal"=w265:bool)  [unwired: 1 in, 5 out]
            n104 = case shown="False" w265 {
              tunnel: [w274 w277] -> w264
              tunnel: w263 -> [w270 w276]
              tunnel: [w269 w276] -> w262
              frame False {
                n105 = Get Date/Time In Seconds() -> (seconds since 1Jan1904=w272:timestamp)
                n106 = call "Convert Data To API String Arguments.vim"("error in (no error)"=w270, "data"=w272) -> ("error out"=w269:errorcluster, "String"=w271:string)  [unwired: 6 in]
                n107 = call-poly <userlib>:"Build Message with Arguments++.vi"("State with Arguments"="API: RESUME", "Arguments (\"\")"=w271, "Target Module (\"\")"="Game Engine" ("Target Module (\"\")")) -> ("State with Arguments out"=w274:string)  [unwired: 12 in]
              }
              frame True {
                n108 = call-poly <userlib>:"Build Message with Arguments++.vi"("State with Arguments"="API: PAUSE", "Target Module (\"\")"="Game Engine" ("Target Module (\"\")")) -> ("State with Arguments out"=w277:string)  [unwired: 13 in]
              }
            }
            n109 = call <vilib>:"Add State(s) to Queue__JKI_lib_State_Machine.vi"("State(s) in Front (\"\")"=w264, "State(s) in (\"\")"=w266) -> ("States Out"=w267:string)  [unwired: 13 in]
          }
          event "save": Value Change {
            n110 = event-data() -> ()  [unwired: 1 in, 4 out]
            n111 = Unbundle By Name(w291) -> ("timeseq.SEQ"=w285:i32[])
            n112 = call "Convert Data To API String Arguments.vim"("error in (no error)"=w290, "data"=w285) -> ("error out"=w288:errorcluster, "String"=w289:string)  [unwired: 6 in]
            n113 = call <userlib>:"CSM - Wait and Send Message for Reply.vi"("State"="API: SAVE", "Current Module(\"\" to generate a ID)"=w281, "Arguments (\"\")"=w289, "Target Module"="Archive", "Error In (no error)"=w288) -> ("Response"=w286:string, "error out"=w282:errorcluster)  [unwired: 8 in, 1 out]
            n114 = case shown="\"Y\", Default" w286 {
              tunnel: w282 -> [w293 w295]
              tunnel: w281 -> [_ w298]
              tunnel: [w293 w297] -> w280
              frame "False" {
              }
              frame "Y", Default {
                n115 = property on="pause" class="Bool (strict)"(error in=w295) -> (error out=w294:errorcluster, "Value"=w296:bool)  [unwired: 1 in, 1 out]
                n116 = case shown="True" w296 {
                  tunnel: w294 -> [w303 w316]
                  tunnel: w298 -> [w302 _]
                  tunnel: [w300 w316] -> w297
                  frame False {
                    n117 = One Button Dialog(message="SAVE SUCCESS") -> (true=w299:bool)  [unwired: 1 in]
                    n118 = call <userlib>:"CSM - Post Message.vi"("Current Module(\"\" to generate a ID)"=w302, "Error In (no error)"=w303, "Target Module"="Game Engine" ("Target Module (\"\")"), "State"="API: PAUSE" ("State with Arguments")) -> ("error out"=w301:errorcluster)  [unwired: 7 in]
                    n119 = case shown="False" w299 {
                      tunnel: w302 -> [_ w311]
                      tunnel: w301 -> [w307 w310]
                      tunnel: [w307 w308] -> w300
                      frame False {
                      }
                      frame True {
                        n120 = Get Date/Time In Seconds() -> (seconds since 1Jan1904=w315:timestamp)
                        n121 = call "Convert Data To API String Arguments.vim"("error in (no error)"=w310, "data"=w315) -> ("error out"=w309:errorcluster, "String"=w312:string)  [unwired: 6 in]
                        n122 = call <userlib>:"CSM - Post Message.vi"("Current Module(\"\" to generate a ID)"=w311, "Error In (no error)"=w309, "Target Module"="Game Engine" ("Target Module (\"\")"), "Arguments (\"\")"=w312, "State"="API: RESUME" ("State with Arguments")) -> ("error out"=w308:errorcluster)  [unwired: 6 in]
                      }
                    }
                  }
                  frame True {
                    n123 = One Button Dialog(message="SAVE SUCCESS") -> ()  [unwired: 1 in, 1 out]
                  }
                }
              }
            }
            n124 = call <vilib>:"Add State(s) to Queue__JKI_lib_State_Machine.vi"("State(s) in (\"\")"=w283) -> ("States Out"=w284:string)  [unwired: 14 in]
          }
          event "exit2": Value Change {
            n125 = event-data() -> ()  [unwired: 1 in, 4 out]
            n126 = Unbundle By Name(w325) -> ("score"=w324:i32, "Tab Control"=w318:refnum<vi>)
            n127 = call "Convert Data To API String Arguments.vim"("error in (no error)"=w322, "data"=w324) -> ("error out"=w321:errorcluster, "String"=w323:string)  [unwired: 6 in]
            n128 = call <vilib>:"Build State String with Arguments__JKI_lib_State_Machine.vi"("Arguments (\"\")"=w323, "State"="GAMEEXIT") -> ("State with Arguments"=w327:string)  [unwired: 4 in]
            n129 = property class="TabCtl (strict)"(reference=w318, error in=w321, "Value"=Control_2."Page 2" ("Tab Control")) -> (error out=w320:errorcluster)  [unwired: 1 out]
            n130 = call <userlib>:"CSM - Broadcast Status Change.vi"("Status with Arguments"=w327, "State Queue"=w329) -> ("Remaining States"=w328:string)  [unwired: 13 in]
          }
          event "Boolean1": Value Change {
            n131 = event-data() -> ()  [unwired: 1 in, 6 out]
            n132 = call-poly <userlib>:"Build Message with Arguments++.vi"("State with Arguments"="API: TAP" ("State"), "Arguments (\"\")"="1" ("Arguments (\"\")"), "Target Module (\"\")"="Game Engine" ("Target Module")) -> ("State with Arguments out"=w334:string)  [unwired: 12 in]
            n133 = flat-sequence {
              tunnel: w332 -> [w341]
              tunnel: [w340] -> w331
              frame #0 {
                n134 = Wait (ms)(milliseconds to wait=u32 100) -> ()  [unwired: 1 out]
              }
              frame #1 {
                n135 = property class="Bool (strict)"(reference=w341, "Value"=FALSE ("Boolean1")) -> (error out=w340:errorcluster)  [unwired: 1 in, 1 out]
              }
            }
            n136 = call <vilib>:"Add State(s) to Queue__JKI_lib_State_Machine.vi"("State(s) in Front (\"\")"=w334, "State(s) in (\"\")"=w335) -> ("States Out"=w336:string)  [unwired: 13 in]
            n137 = Unbundle By Name(w333) -> ("Boolean1"=w332:refnum<vi>)
          }
          event "Boolean 2": Value Change {
            n138 = event-data() -> ()  [unwired: 1 in, 6 out]
            n139 = call-poly <userlib>:"Build Message with Arguments++.vi"("State with Arguments"="API: TAP" ("State"), "Arguments (\"\")"="2" ("Arguments (\"\")"), "Target Module (\"\")"="Game Engine" ("Target Module")) -> ("State with Arguments out"=w346:string)  [unwired: 12 in]
            n140 = flat-sequence {
              tunnel: [w354] -> w345
              tunnel: w343 -> [w353]
              frame #0 {
                n141 = Wait (ms)(milliseconds to wait=u32 100) -> ()  [unwired: 1 out]
              }
              frame #1 {
                n142 = property class="Bool (strict)"(reference=w353, "Value"=FALSE ("Boolean 2")) -> (error out=w354:errorcluster)  [unwired: 1 in, 1 out]
              }
            }
            n143 = Unbundle By Name(w344) -> ("Boolean 2"=w343:refnum<vi>)
            n144 = call <vilib>:"Add State(s) to Queue__JKI_lib_State_Machine.vi"("State(s) in Front (\"\")"=w346, "State(s) in (\"\")"=w347) -> ("States Out"=w348:string)  [unwired: 13 in]
          }
          event "Boolean 3": Value Change {
            n145 = event-data() -> ()  [unwired: 1 in, 6 out]
            n146 = call-poly <userlib>:"Build Message with Arguments++.vi"("State with Arguments"="API: TAP" ("State"), "Arguments (\"\")"="3" ("Arguments (\"\")"), "Target Module (\"\")"="Game Engine" ("Target Module")) -> ("State with Arguments out"=w359:string)  [unwired: 12 in]
            n147 = flat-sequence {
              tunnel: w357 -> [w367]
              tunnel: [w366] -> w356
              frame #0 {
                n148 = Wait (ms)(milliseconds to wait=u32 100) -> ()  [unwired: 1 out]
              }
              frame #1 {
                n149 = property class="Bool (strict)"(reference=w367, "Value"=FALSE ("Boolean1")) -> (error out=w366:errorcluster)  [unwired: 1 in, 1 out]
              }
            }
            n150 = Unbundle By Name(w358) -> ("Boolean 3"=w357:refnum<vi>)
            n151 = call <vilib>:"Add State(s) to Queue__JKI_lib_State_Machine.vi"("State(s) in Front (\"\")"=w359, "State(s) in (\"\")"=w360) -> ("States Out"=w361:string)  [unwired: 13 in]
          }
          event "Boolean 4": Value Change {
            n152 = event-data() -> ()  [unwired: 1 in, 6 out]
            n153 = call-poly <userlib>:"Build Message with Arguments++.vi"("State with Arguments"="API: TAP" ("State"), "Arguments (\"\")"="4" ("Arguments (\"\")"), "Target Module (\"\")"="Game Engine" ("Target Module")) -> ("State with Arguments out"=w372:string)  [unwired: 12 in]
            n154 = call <vilib>:"Add State(s) to Queue__JKI_lib_State_Machine.vi"("State(s) in Front (\"\")"=w372, "State(s) in (\"\")"=w373) -> ("States Out"=w374:string)  [unwired: 13 in]
            n155 = Unbundle By Name(w371) -> ("Boolean 4"=w370:refnum<vi>)
            n156 = flat-sequence {
              tunnel: w370 -> [w381]
              tunnel: [w379] -> w369
              frame #0 {
                n157 = Wait (ms)(milliseconds to wait=u32 100) -> ()  [unwired: 1 out]
              }
              frame #1 {
                n158 = property class="Bool (strict)"(reference=w381, "Value"=FALSE ("Boolean1")) -> (error out=w379:errorcluster)  [unwired: 1 in, 1 out]
              }
            }
          }
          event User Event {
            # "#CSM \"New State Notifier Event\"\nThis user event is used to break out CSM from waiting in the event structure, to process the next state from external. DO NOT place any code here unless you really need to."
            n159 = event-data() -> ()  [unwired: 1 in, 1 out]
          }
          event Panel Close? {
            # "#CSM Discard Panel Close?\nDiscard the event because we'll close the front panel ourselves in Macro: Exit"
            n160 = event-data() -> ()  [unwired: 1 in, 1 out]
            n161 = call <vilib>:"Add State(s) to Queue__JKI_lib_State_Machine.vi"("State(s) in Front (\"\")"="Macro: Exit", "State(s) in (\"\")"=w388) -> ("States Out"=w387:string)  [unwired: 13 in]
            n162 = event-data("Discard?"=TRUE) -> ()  [unwired: 1 in, 1 out]
          }
          event "Stop": Value Change {
            n163 = event-data() -> ()  [unwired: 1 in, 6 out]
            n164 = call <vilib>:"Add State(s) to Queue__JKI_lib_State_Machine.vi"("State(s) in Front (\"\")"=" Macro: Exit" ("State(s) in Front (\"\")"), "State(s) in (\"\")"=w390) -> ("States Out"=w391:string)  [unwired: 13 in]
            n165 = call <userlib>:"CSM - Broadcast Status Change.vi"("Status with Arguments"="EXIT", "State Queue"=w391) -> ("Remaining States"=w392:string)  [unwired: 13 in]
          }
        }
      }
      frame "CSM Documentation" {
        # "#CSM Documentation"
        # "#CSM State Syntax\n\n// Comment line, all text to the right of “//” will be ignored\n// Local Message Example\nDoSth: DoA >> Arguments\n\n// Sync Call Example\nAPI: xxxx >> Arguments -@ TargetModule\n\n// Async Call Example\nAPI: xxxx >> Arguments -> TargetModule\n\n// Async Call without Reply Example\nAPI: xxxx >> Arguments ->| TargetModule\n\n// Broadcast normal status:\nStatus >> StatusArguments  -><status>\n\n// Broadcast Interrupt status:\nInterrupt >> StatusArguments  -><interrupt>\n\n// Register Source Module's status to Handler Module\nStatus@Source Module >> Handler Module@Handler Module -><register>\n\n// Unegister Source Module's status\nStatus@Source Module >> Handler Module -><unregister>"
        # "#CSM README FIRST\n\nCommunicable State Machine(CSM) is a LabVIEW application framework that builds upon JKI State Machine(JKISM). It follows the pattern of JKISM and extends the keywords to describe message communication between modules, including concepts such as Sync-Message, Async-Message, Subscription/Unsubscription of status - essential elements for creating reusable code modules. For more information, please visit the CSM wiki: https://nevstop-lab.github.io/CSM-Wiki/\n\nFor instructions on JKI State Machine, visit: \n    http://jki.net/state-machine/\nFor information about CSM, visit: \n    https://github.com/NEVSTOP-LAB"
        # "#CSM \"Documentation\"\nCase for holding CSM Documenation"
      }
      frame "---------- Core ----------" {
        # "#CSM \"Category Seperator\"\nDo not put any code in this frame."
        n166 = call <vilib>:"Add State(s) to Queue__JKI_lib_State_Machine.vi"("State(s) in (\"\")"=w402) -> ("States Out"=w401:string)  [unwired: 14 in]
      }
      frame Default {
        # "#CSM \"Default\"\nthis is used to capture unhandled states and typos"
        n167 = call <userlib>:"CSM Unhandled State Error.vi"("error in (no error)"=w404, "Current State"=w405, "CSM Name"=w406) -> ("error out"=w403:errorcluster)  [unwired: 8 in]
        n168 = call <vilib>:"Add State(s) to Queue__JKI_lib_State_Machine.vi"("State(s) in (\"\")"=w411) -> ("States Out"=w410:string)  [unwired: 14 in]
      }
      frame "VI Reference" {
        n169 = Unbundle By Name(w416) -> ("Core"=w414:T8)
        n170 = Unbundle By Name(w414) -> ("Current VI Reference"=w413:refnum<vi>)
        n171 = call <userlib>:"CSM - Convert Data to HexStr.vi"("Variant"=w413) -> ("HEX String (0-9,A-F)"=w412:string)  [unwired: 8 in]
      }
      frame "Error Handler" {
        # "#CSM Disable this error dialog if you need"
        # "#CSM \"Error Handler\"\nYou can also output any states to clean-up after errors occur"
        # "Clear error"
        n172 = case shown="Error" w428 {
          selector: w428 -> [_ w439]
          tunnel: [w435 w438] -> w425
          tunnel: w424 -> [w435 w440]
          tunnel: [w434 w439] -> w423
          tunnel: w422 -> [w436 _]
          tunnel: w421 -> [_ _]
          tunnel: w420 -> [_ _]
          frame No Error {
            n173 = call <userlib>:"CSM - Convert Argument to Error.vi"("Argument"=w436) -> ("error"=w434:errorcluster)  [unwired: 4 in]
            n174 = flat-sequence {
              frame #0 {
                # "#CSM External Error Handler Case\nUsually, it's because This CSM register others' \"Error Occurred\" status with \"Error Handler\". If other CSM have any error, the error will be passed here for central handling."
              }
            }
          }
          frame Error {
            # "#CSM Internal Error Handler Case \nIf any error Occurred, \"Error Occurred\" \nstatus update will be broadcasted to system.\nParameter is Error Cluster."
            n175 = call <userlib>:"CSM - Convert Error to Argument.vi"("error in (no error)"=w439) -> ("Arguments"=w442:string)  [unwired: 4 in]
            n176 = call <vilib>:"Build State String with Arguments__JKI_lib_State_Machine.vi"("Arguments (\"\")"=w442, "State"="Error Occurred" ("Status with Arguments")) -> ("State with Arguments"=w441:string)  [unwired: 4 in]
            n177 = call <userlib>:"CSM - Broadcast Status Change.vi"("Status with Arguments"=w441, "State Queue"=w440) -> ("Remaining States"=w437:string)  [unwired: 13 in]
            n178 = call <vilib>:"Add State(s) to Queue__JKI_lib_State_Machine.vi"("State(s) in (\"\")"=w437) -> ("States Out"=w438:string)  [unwired: 14 in]
          }
        }
        n179 = disable-structure shown="Enabled" {
          disable-tunnel: w423 -> [w432 w433]
          frame Enabled {
            # "Unhandled Error -- Display it"
            n180 = call <vilib>:"General Error Handler.vi"("error in (no error)"=w432) -> ()  [unwired: 10 in, 5 out]
          }
          frame Disabled {
            n181 = call <vilib>:"Clear Errors.vi"("error in (no error)"=w433) -> ()  [unwired: 5 in, 2 out]
          }
        }
        n182 = call <vilib>:"Add State(s) to Queue__JKI_lib_State_Machine.vi"("State(s) in Front (\"\")"="// Post Error States", "State(s) in (\"\")"=w425) -> ("States Out"=w426:string)  [unwired: 13 in]
      }
      frame "Critical Error" {
        # "#CSM \"Critical Error\"\nWhen any un-recoverable error occurs, CSM goes into this case."
        # "#CSM Stop in Critical Error\nWhen Critical Error occurs, Stop the loop immediately. Do NOT change this unless you fully understand the impact."
        n183 = call <userlib>:"CSM Critical Error.vi"("error in (no error)"=w445, "Arugments(as Reason)"=w447, "CSM Name"=w446) -> ("error out"=w444:errorcluster)  [unwired: 8 in]
        n184 = call <vilib>:"Add State(s) to Queue__JKI_lib_State_Machine.vi"("State(s) in (\"\")"=w451) -> ("States Out"=w450:string)  [unwired: 14 in]
      }
      frame "Target Timeout Error" {
        # "#CSM \"Target Timeout Error\"\nWhen This CSM could not get the sync-call response in time, This CSM goes into this case."
        n185 = call <userlib>:"CSM Target Timeout Error.vi"("error in (no error)"=w455, "Arguments(as CSM Name)"=w454) -> ("error out"=w453:errorcluster)  [unwired: 9 in]
        n186 = call <vilib>:"Add State(s) to Queue__JKI_lib_State_Machine.vi"("State(s) in (\"\")"=w459) -> ("States Out"=w458:string)  [unwired: 14 in]
      }
      frame "Target Error" {
        # "#CSM \"Target Error\"\nWhen This CSM try to communicate with an un-existed CSM, This CSM goes into this case."
        n187 = call <userlib>:"CSM Target Error.vi"("error in (no error)"=w461, "Arguments(as CSM Name)"=w462) -> ("error out"=w460:errorcluster)  [unwired: 9 in]
        n188 = call <vilib>:"Add State(s) to Queue__JKI_lib_State_Machine.vi"("State(s) in (\"\")"=w466) -> ("States Out"=w465:string)  [unwired: 14 in]
      }
      frame "Async Response", "Response" {
        # "#CSM \"Async Response\"\nHandle Async-call Response (\"Async Response\" for ->)"
        # "#CSM \"Response\"\nHandle Sync-call Response (\"Response\" for -@)"
        n189 = Unbundle(w472) -> ("‘State"=w469:string, "’Arguments"=w468:string, "’Error"=w467:errorcluster)
        n190 = case shown="Default" w469 {
          tunnel: [w479] -> w477
          tunnel: w476 -> [w480]
          tunnel: [w482] -> w475
          tunnel: w474 -> [w482]
          tunnel: [w481] -> w473
          tunnel: w467 -> [w481]
          tunnel: w471 -> [_]
          tunnel: w470 -> [_]
          tunnel: w468 -> [_]
          frame Default {
            # "#CSM Response Comments\nAfter Message is executed, CSM goes to this state for receive the response.\n    For Async Message(->), \"Async Response\" is used. This CSM will goes to \"Async Message Posted\" immediately and receive the \"Async Response\" after the callee finishes the message.\n    For Sync Message(@),  This CSM will wait until the message is done and immediately goes to \"Response\""
            n191 = call <vilib>:"Add State(s) to Queue__JKI_lib_State_Machine.vi"("State(s) in (\"\")"=w480) -> ("States Out"=w479:string)  [unwired: 14 in]
          }
        }
      }
      frame "Async Message Posted" {
        # "#CSM \"Async Message Posted\"\nAfter Async Message is posted (-> or ->| ), CSM goes to this state for post-action.\nYou can use Argument - State to tell which Async Message is called."
      }
      frame "Initialize Core Data" {
        # "#CSM \"Initialize Core Data\"\nThis is used to determine panel behavior on exit"
        # "originally closed?"
        # "exe?"
        # "If panel starts closed or is an EXE, then close it when we exit"
        n192 = property class="VI"() -> ("FP.State"=w489:T4)  [unwired: 2 in, 2 out]
        n193 = property class="App"() -> ("App.Kind"=w495:T5)  [unwired: 2 in, 2 out]
        n194 = control-ref of="Current VI Reference"() -> (w490:refnum<vi>)
        n195 = Equal?(x=w489, y=T4."Closed" ("Front Panel Window:State")) -> (x = y?=w487:bool)
        n196 = Equal?(x=w495, y=T5."Run Time System" ("Application:Kind")) -> (x = y?=w493:bool)
        n197 = Or(x=w487, y=w493) -> (x .or. y?=w491:bool)
        n198 = Bundle By Name(cluster=w492, "Core.Current VI Reference"=w490, "Core.Close Panel on Exit?"=w491) -> (w496:T7)
        n199 = call <vilib>:"Add State(s) to Queue__JKI_lib_State_Machine.vi"("State(s) in (\"\")"=w498) -> ("States Out"=w497:string)  [unwired: 14 in]
      }
      frame "Exit" {
        # "#CSM \"Exit\"\nCase for exiting the loop. No errors that occur here will be handled."
        n200 = call <vilib>:"Add State(s) to Queue__JKI_lib_State_Machine.vi"("State(s) in (\"\")"=w503) -> ("States Out"=w502:string)  [unwired: 14 in]
      }
      frame "---------- Data ----------" {
        # "#CSM \"Category Seperator\"\nDo not put any code in this frame."
        n201 = call <vilib>:"Add State(s) to Queue__JKI_lib_State_Machine.vi"("State(s) in (\"\")"=w507) -> ("States Out"=w506:string)  [unwired: 14 in]
      }
      frame "Data: Initialize" {
        w510 = cluster{"time":i32, "SEQ":i32[]} {"time"=10, "SEQ"=[]}  # timeseq
        w511 = 0.0  # start time
        w517 = string[][] []  # rank
        w521 = 0  # score
        w522 = cluster{"username":string, "password":string} {"username"="", "password"=""}  # ID
        w524 = T8 {"Current VI Reference"=refnum, "Close Panel on Exit?"=FALSE}  # Core
        # "#CSM  do not delete - used by framework"
        # "#CSM \"Data: Initialize\"\nInitialize the shift-register data, here.\n(data names are defined by what you wire into the bundle function)"
        n202 = call <vilib>:"Application Directory.vi"() -> ("Application Directory"=w520:path)
        n203 = Build Path(base path=w520, name or relative path=path "rank.ini") -> (appended path=w518:path)
        n204 = control-ref of="Countdown"() -> (w509:refnum<vi>)
        n205 = control-ref of="Boolean 2"() -> (w516:refnum<vi>)
        n206 = control-ref of="Boolean 4"() -> (w515:refnum<vi>)
        n207 = control-ref of="Boolean 3"() -> (w514:refnum<vi>)
        n208 = control-ref of="start2"() -> (w512:refnum<vi>)
        n209 = control-ref of="Boolean1"() -> (w513:refnum<vi>)
        n210 = control-ref of="Tab Control"() -> (w508:refnum<vi>)
        n211 = Bundle("Tab Control"=w508, "start2"=w512, "Boolean1"=w513, "Boolean 3"=w514, "Boolean 4"=w515, "Boolean 2"=w516, "Core"=w524, "rank"=w517, "ID"=w522, "score"=w521, "timeseq"=w510, "appended path"=w518, "start time"=w511, "Countdown"=w509) -> (w525:T7)  [unwired: 1 in]
        n212 = call <vilib>:"Add State(s) to Queue__JKI_lib_State_Machine.vi"("State(s) in (\"\")"=w527) -> ("States Out"=w526:string)  [unwired: 14 in]
      }
      frame "Data: Cleanup" {
        # "#CSM \"Data: Cleanup\"\nCleanup any data and references, here.\n(this is called automatically, by the Macro: Exit)"
        n213 = Unbundle By Name(w529) -> ("Core.Current VI Reference"=w531:refnum<vi>)
        n214 = Close Reference(reference=w531) -> (error out=w530:errorcluster)  [unwired: 1 in]
        n215 = call <vilib>:"Add State(s) to Queue__JKI_lib_State_Machine.vi"("State(s) in (\"\")"=w533) -> ("States Out"=w532:string)  [unwired: 14 in]
      }
      frame "---------- Events ----------" {
        # "#CSM \"Category Seperator\"\nDo not put any code in this frame."
        n216 = call <vilib>:"Add State(s) to Queue__JKI_lib_State_Machine.vi"("State(s) in (\"\")"=w537) -> ("States Out"=w536:string)  [unwired: 14 in]
      }
      frame "Events: Register" {
        # "#CSM \"Events: Register\"\nRegister user event. New Message Event is registered to break CSM waiting in event structure by default."
        # "#CSM Register New Message Event\nRegister message event to break Waiting in Event structure."
        n217 = call <userlib>:"CSM - Get New State Notifier Event.vi"("Name(\"\" to use uuid) in"=w541) -> ("Error out"=w539:errorcluster, "New State Notifier Event"=w540:refnum<user-event>)  [unwired: 9 in]
        n218 = register-events(error in=w539, w540) -> (reference out=w542:refnum<event-registration>, error out=w538:errorcluster)  [unwired: 1 in]
      }
      frame "Events: Unregister" {
        # "#CSM \"Events: Unregister\"\nUnregister user event."
        n219 = Unregister For Events(event registration refnum=w545) -> (error out=w546:errorcluster)  [unwired: 1 in]
      }
      frame "---------- UI ----------" {
        # "#CSM \"Category Seperator\"\nDo not put any code in this frame."
        n220 = call <vilib>:"Add State(s) to Queue__JKI_lib_State_Machine.vi"("State(s) in (\"\")"=w552) -> ("States Out"=w551:string)  [unwired: 14 in]
      }
      frame "UI: Initialize" {
        w559 = 0.0 ("time")
        w566 = FALSE ("pause")
        w565 = "" ("username")
        # "#CSM \"UI: Initialize\"\nInitialize the User Interface, here.\n(this is called automatically, by the Macro: Init)"
        n221 = Unbundle By Name(w574) -> ("Countdown"=w560:refnum<vi>, "Boolean1"=w570:refnum<vi>, "Boolean 3"=w571:refnum<vi>, "Boolean 4"=w572:refnum<vi>, "Boolean 2"=w573:refnum<vi>, "Tab Control"=w553:refnum<vi>)
        n222 = property class="TabCtl (strict)"(reference=w553, error in=w557, "Value"=Control_2."Page 1" ("Tab Control")) -> (error out=w556:errorcluster)  [unwired: 1 out]
        n223 = property class="DigNum (strict)"(reference=w560, error in=w556, "Value"=w559) -> (error out=w555:errorcluster)  [unwired: 1 out]
        n224 = property class="Bool (strict)"(reference=w573, error in=w555, "Value"=w566) -> (error out=w569:errorcluster)  [unwired: 1 out]
        n225 = property class="Bool (strict)"(reference=w572, error in=w569, "Value"=w566) -> (error out=w568:errorcluster)  [unwired: 1 out]
        n226 = property class="Bool (strict)"(reference=w571, error in=w568, "Value"=w566) -> (error out=w567:errorcluster)  [unwired: 1 out]
        n227 = property class="Bool (strict)"(reference=w570, error in=w567, "Value"=w566) -> (error out=w564:errorcluster)  [unwired: 1 out]
        n228 = property on="username" class="Str"(error in=w564, "Value"=w565) -> (error out=w563:errorcluster)  [unwired: 1 in, 1 out]
        n229 = property on="password" class="Str"(error in=w563, "Value"=w565) -> (error out=w562:errorcluster)  [unwired: 1 in, 1 out]
        n230 = property on="pause" class="Bool (strict)"(error in=w562, "Value"=w566) -> (error out=w561:errorcluster)  [unwired: 1 in, 1 out]
        n231 = property on="time" class="DigNum (strict)"(error in=w561, "Value"=w559) -> (error out=w554:errorcluster)  [unwired: 1 in, 1 out]
        n232 = call <vilib>:"Add State(s) to Queue__JKI_lib_State_Machine.vi"("State(s) in (\"\")"=w577) -> ("States Out"=w576:string)  [unwired: 14 in]
      }
      frame "UI: Cursor Set" {
        # "Argument"
        # "#CSM \"UI: Cursor Set\"\nSet and Unset Cursor Busy.\n(Usage: \"UI: Cursor Set >> Busy|Idle\")"
        n233 = disable-structure shown="Default" {
          disable-tunnel: [w585 w588] -> w580
          disable-tunnel: w579 -> [w584 _]
          frame condition #0 (active) {
            n234 = case shown="\"Idle\", Default" w584 {
              tunnel: [w586 w587] -> w585
              frame "Idle", Default {
                n235 = call <vilib>:"Unset Busy.vi"() -> ("error out"=w586:errorcluster)  [unwired: 11 in]
              }
              frame "Busy" {
                n236 = call <vilib>:"Set Busy.vi"() -> ("error out"=w587:errorcluster)  [unwired: 10 in, 1 out]
              }
            }
          }
          frame condition #1 {
          }
        }
        n237 = call <vilib>:"Add State(s) to Queue__JKI_lib_State_Machine.vi"("State(s) in (\"\")"=w583) -> ("States Out"=w582:string)  [unwired: 14 in]
      }
      frame "UI: Front Panel State" {
        # "Argument"
        # "#CSM \"UI: Front Panel State\"\nSet Front Panel Open or Closed\n(Usage: \"UI: Front Panel State >> Open|Close\")"
        n238 = Unbundle By Name(w594) -> ("Core.Current VI Reference"=w591:refnum<vi>)
        n239 = case shown="\"Hidden\", \"Hide\"" w593 {
          tunnel: [w603 w616 w627 w639 w651] -> w590
          tunnel: w591 -> [w602 w614 w626 w638 w650]
          frame "Open", "Standard", Default {
            w597 = T4."Standard" ("State")
            n240 = property class="VI"(reference=w602) -> (reference out=w600:refnum<vi>, error out=w601:errorcluster, "FP.State"=w599:T4)  [unwired: 1 in]
            n241 = Not Equal?(x=w599, y=w597) -> (x != y?=w598:bool)
            n242 = case shown="True" w598 {
              tunnel: [w607 w609] -> w603
              tunnel: w601 -> [w606 w609]
              tunnel: w600 -> [w605 _]
              tunnel: w597 -> [w604 _]
              frame True {
                n243 = invoke class="VI" method="FP.Open"(reference=w605, error in=w606, "Activate"=TRUE, "State"=w604) -> (error out=w607:errorcluster)  [unwired: 1 in, 4 out]
              }
              frame False {
              }
            }
          }
          frame "Close", "Closed" {
            n244 = property class="VI"(reference=w614) -> (reference out=w613:refnum<vi>, error out=w615:errorcluster, "FP.State"=w611:T4)  [unwired: 1 in]
            n245 = Not Equal?(x=w611, y=T4."Closed" ("Front Panel Window:State")) -> (x != y?=w610:bool)
            n246 = case shown="True" w610 {
              tunnel: [w617 w620] -> w616
              tunnel: w615 -> [w617 w619]
              tunnel: w613 -> [_ w618]
              frame False {
              }
              frame True {
                n247 = invoke class="VI" method="FP.Close"(reference=w618, error in=w619) -> (error out=w620:errorcluster)  [unwired: 1 in, 2 out]
              }
            }
          }
          frame "Hidden", "Hide" {
            w621 = T4."Hidden" ("State")
            n248 = property class="VI"(reference=w626) -> (reference out=w624:refnum<vi>, error out=w625:errorcluster, "FP.State"=w623:T4)  [unwired: 1 in]
            n249 = Not Equal?(x=w623, y=w621) -> (x != y?=w622:bool)
            n250 = case shown="True" w622 {
              tunnel: [w631 w632] -> w627
              tunnel: w625 -> [w630 w632]
              tunnel: w624 -> [w629 _]
              tunnel: w621 -> [w628 _]
              frame True {
                n251 = invoke class="VI" method="FP.Open"(reference=w629, error in=w630, "State"=w628) -> (error out=w631:errorcluster)  [unwired: 2 in, 4 out]
              }
              frame False {
              }
            }
          }
          frame "Minimize", "Minimized" {
            w633 = T4."Minimized" ("State")
            n252 = property class="VI"(reference=w638) -> (reference out=w636:refnum<vi>, error out=w637:errorcluster, "FP.State"=w635:T4)  [unwired: 1 in]
            n253 = Not Equal?(x=w635, y=w633) -> (x != y?=w634:bool)
            n254 = case shown="True" w634 {
              tunnel: [w643 w644] -> w639
              tunnel: w637 -> [w642 w644]
              tunnel: w636 -> [w641 _]
              tunnel: w633 -> [w640 _]
              frame True {
                n255 = invoke class="VI" method="FP.Open"(reference=w641, error in=w642, "State"=w640) -> (error out=w643:errorcluster)  [unwired: 2 in, 4 out]
              }
              frame False {
              }
            }
          }
          frame "Maximize", "Maximized" {
            w645 = T4."Maximized" ("State")
            n256 = property class="VI"(reference=w650) -> (reference out=w648:refnum<vi>, error out=w649:errorcluster, "FP.State"=w647:T4)  [unwired: 1 in]
            n257 = Not Equal?(x=w647, y=w645) -> (x != y?=w646:bool)
            n258 = case shown="True" w646 {
              tunnel: [w655 w656] -> w651
              tunnel: w649 -> [w654 w656]
              tunnel: w648 -> [w653 _]
              tunnel: w645 -> [w652 _]
              frame True {
                n259 = invoke class="VI" method="FP.Open"(reference=w653, error in=w654, "State"=w652) -> (error out=w655:errorcluster)  [unwired: 2 in, 4 out]
              }
              frame False {
              }
            }
          }
        }
        n260 = invoke class="VI" method="FP.Center"(reference=w591, error in=w590) -> (error out=w589:errorcluster)  [unwired: 1 in, 2 out]
        n261 = call <vilib>:"Add State(s) to Queue__JKI_lib_State_Machine.vi"("State(s) in (\"\")"=w596) -> ("States Out"=w595:string)  [unwired: 14 in]
      }
      frame "---------- Macro ----------" {
        # "#CSM \"Category Seperator\"\nDo not put any code in this frame."
        n262 = call <vilib>:"Add State(s) to Queue__JKI_lib_State_Machine.vi"("State(s) in (\"\")"=w660) -> ("States Out"=w659:string)  [unwired: 14 in]
      }
      frame "Macro: Initialize" {
        w662 = "Data: Initialize\nInitialize Core Data\nEvents: Register\nUI: Initialize\nUI: Front Panel State >> Open"  # Data: Initialize Initialize Core Data Events: Register UI: Initialize UI: Front Panel State >> Open
        # "#CSM \"Macro: Initialize\"\nInitialization Macro (This is called once, when the VI starts)"
        n263 = call <vilib>:"Add State(s) to Queue__JKI_lib_State_Machine.vi"("State(s) in Front (\"\")"=w662, "State(s) in (\"\")"=w665) -> ("States Out"=w664:string)  [unwired: 13 in]
      }
      frame "Macro: Exit" {
        # "#CSM \"Macro: Exit\"\nExit Macro (This is called once, when the VI exits)"
        n264 = Unbundle By Name(w674) -> ("Core.Close Panel on Exit?"=w673:bool)
        n265 = Select(t="UI: Front Panel State >> Close", s=w673, f="") -> (s? t:f=w670:string)
        n266 = call <vilib>:"Add State(s) to Queue__JKI_lib_State_Machine.vi"("State(s) in Front (\"\")"="//Exit Sub-Modules ", "State(s) in (\"\")"=w670, "State(s) at Back (\"\")"="Data: Cleanup\nEvents: Unregister\nExit") -> ("States Out"=w668:string)  [unwired: 12 in]
        n267 = call <vilib>:"Add State(s) to Queue__JKI_lib_State_Machine.vi"("State(s) in Front (\"\")"=w668, "State(s) in (\"\")"=w676) -> ("States Out"=w675:string)  [unwired: 13 in]
      }
      frame "---------- API ----------" {
        # "#CSM \"Category Seperator\"\nDo not put any code in this frame."
      }
      frame "API: BLINK" {
        # "#CSM \"Category Seperator\"\nDo not put any code in this frame."
        n268 = call "Convert API String Arguments to Data.vim"("Type"=i32[] [], "String"=w692) -> ("error"=w684:errorcluster, "Data"=w690:i32[])  [unwired: 6 in]
        n269 = Bundle By Name(cluster=w691, "timeseq.SEQ"=w690) -> (w686:T7)
        n270 = Unbundle By Name(w686) -> ("Boolean1"=w685:refnum<vi>, "Boolean 2"=w681:refnum<vi>, "Boolean 3"=w680:refnum<vi>, "Boolean 4"=w682:refnum<vi>)
        n271 = for {
          tunnel: w690 -> [w700] mode=indexing
          tunnel: w685 -> [w699]
          tunnel: bool[] [TRUE, FALSE] -> [w698]
          tunnel: w682 -> [w697]
          tunnel: w681 -> [w696]
          tunnel: w680 -> [w695]
          n272 = case shown="4, Default" w700 {
            tunnel: w699 -> [_ _ _ w717]
            tunnel: w698 -> [w702 w707 w712 w716]
            tunnel: w697 -> [w701 _ _ _]
            tunnel: w696 -> [_ w706 _ _]
            tunnel: w695 -> [_ _ w711 _]
            frame 4, Default {
              n273 = for {
                tunnel: w702 -> [w703] mode=indexing
                tunnel: w701 -> [w704]
                n274 = property class="Bool (strict)"(reference=w704, "Value"=w703) -> ()  [unwired: 1 in, 2 out]
                n275 = Wait (ms)(milliseconds to wait=u32 200) -> ()  [unwired: 1 out]
              }
            }
            frame 2 {
              n276 = for {
                tunnel: w707 -> [w708] mode=indexing
                tunnel: w706 -> [w709]
                n277 = property class="Bool (strict)"(reference=w709, "Value"=w708) -> ()  [unwired: 1 in, 2 out]
                n278 = Wait (ms)(milliseconds to wait=u32 200) -> ()  [unwired: 1 out]
              }
            }
            frame 3 {
              n279 = for {
                tunnel: w712 -> [w714] mode=indexing
                tunnel: w711 -> [w713]
                n280 = property class="Bool (strict)"(reference=w713, "Value"=w714) -> ()  [unwired: 1 in, 2 out]
                n281 = Wait (ms)(milliseconds to wait=u32 200) -> ()  [unwired: 1 out]
              }
            }
            frame 1 {
              n282 = for {
                tunnel: w716 -> [w718] mode=indexing
                tunnel: w717 -> [w719]
                n283 = property class="Bool (strict)"(reference=w719, "Value"=w718) -> ()  [unwired: 1 in, 2 out]
                n284 = Wait (ms)(milliseconds to wait=u32 200) -> ()  [unwired: 1 out]
              }
            }
          }
        }
        n285 = call <vilib>:"Add State(s) to Queue__JKI_lib_State_Machine.vi"("State(s) in Front (\"\")"="Action: ENABLE" ("State(s) in (\"\")"), "State(s) in (\"\")"=w688) -> ("States Out"=w689:string)  [unwired: 13 in]
      }
      frame "API: SHOW" {
        # "#CSM \"Category Seperator\"\nDo not put any code in this frame."
        n286 = call "Convert API String Arguments to Data.vim"("Type"=0.0, "error in (no error)"=w727, "String"=w728) -> ("error"=w726:errorcluster, "Data"=w722:dbl)  [unwired: 5 in]
        "time" <- w722
        n287 = Unbundle By Name(w724) -> ("timeseq.time"=w723:i32)
        n288 = Subtract(x=w723, y=w722) -> (x-y=→"Countdown":dbl)
        n289 = call <vilib>:"Add State(s) to Queue__JKI_lib_State_Machine.vi"("State(s) in (\"\")"=w731) -> ("States Out"=w730:string)  [unwired: 14 in]
      }
      frame "API: PASS" {
        # "#CSM API Example\nCopy/Rename this case for your own API"
        n290 = Unbundle By Name(w734) -> ("timeseq.SEQ"=w745:i32[], "Countdown"=w738:refnum<vi>)
        n291 = property class="DigNum (strict)"(reference=w738, error in=w737, "Value"=0.0) -> (error out=w736:errorcluster)  [unwired: 1 out]
        n292 = Array Size(array=w745) -> (size(s)=w732:i32)
        n293 = call "Convert Data To API String Arguments.vim"("error in (no error)"=w736, "data"=w745) -> ("error out"=w744:errorcluster, "String"=w747:string)  [unwired: 6 in]
        n294 = call-poly <userlib>:"Build Message with Arguments++.vi"("State with Arguments"="API: SEQ", "Arguments (\"\")"=w747, "Target Module (\"\")"="Game Engine" ("Target Module (\"\")")) -> ("State with Arguments out"=w743:string)  [unwired: 12 in]
        n295 = property on="score" class="DigNum (strict)"(error in=w744, "Value"=w732) -> (error out=w741:errorcluster)  [unwired: 1 in, 1 out]
        n296 = property on="time" class="DigNum (strict)"(error in=w741, "Value"=0.0 ("time")) -> (error out=w739:errorcluster)  [unwired: 1 in, 1 out]
        n297 = call <vilib>:"Add State(s) to Queue__JKI_lib_State_Machine.vi"("State(s) in Front (\"\")"="Action: DISABLE" ("State(s) in Front (\"\")"), "State(s) in (\"\")"=w750, "State(s) at Back (\"\")"=w743) -> ("States Out"=w751:string)  [unwired: 12 in]
        n298 = Bundle By Name(cluster=w734, "score"=w732) -> (w733:T7)
        n299 = Wait (ms)(milliseconds to wait=u32 200) -> ()  [unwired: 1 out]
      }
      frame "API: OVER" {
        w754 = 0.0 ("time")
        # "#CSM API Example\nCopy/Rename this case for your own API"
        n300 = Unbundle By Name(w777) -> ("timeseq.SEQ"=w776:i32[], "start2"=w761:refnum<vi>, "Countdown"=w755:refnum<vi>)
        n301 = property class="Bool"(reference=w761, error in=w762, "DisabledEnum"=T3."Enabled" ("Disabled")) -> (error out=w763:errorcluster)  [unwired: 1 out]
        n302 = Array Size(array=w776) -> (size(s)=w775:i32)
        n303 = Bundle By Name(cluster=w777, "score"=0, "timeseq.SEQ"=i32[] [] ("SEQ")) -> (w781:T7)
        n304 = Subtract(x=w775, y=1) -> (x-y=w758:i32)
        n305 = call "Convert Data To API String Arguments.vim"("error in (no error)"=w763, "data"=w758) -> ("error out"=w760:errorcluster, "String"=w767:string)  [unwired: 6 in]
        n306 = Number To Decimal String(number=w758) -> (decimal integer string=w779:string)  [unwired: 1 in]
        n307 = call-poly <userlib>:"Build Message with Arguments++.vi"("State with Arguments"="API: IN", "Arguments (\"\")"=w767, "Target Module (\"\")"="Rank" ("Target Module (\"\")")) -> ("State with Arguments out"=w769:string)  [unwired: 12 in]
        n308 = property on="time" class="DigNum (strict)"(error in=w760, "Value"=w754) -> (error out=w759:errorcluster)  [unwired: 1 in, 1 out]
        n309 = property on="score" class="DigNum (strict)"(error in=w759, "Value"=0 ("y")) -> (error out=w757:errorcluster)  [unwired: 1 in, 1 out]
        n310 = Concatenate Strings("GAME OVER\nYOUR SCORE IS " ("message"), w779) -> (w778:string)
        n311 = property class="DigNum (strict)"(reference=w755, error in=w757, "Value"=w754) -> (error out=w756:errorcluster)  [unwired: 1 out]
        n312 = call <vilib>:"Add State(s) to Queue__JKI_lib_State_Machine.vi"("State(s) in Front (\"\")"=w769, "State(s) in (\"\")"=w770, "State(s) at Back (\"\")"="Action: DISABLE" ("State(s) at Back (\"\")")) -> ("States Out"=w771:string)  [unwired: 12 in]
        n313 = One Button Dialog(message=w778) -> ()  [unwired: 1 in, 1 out]
      }
      frame "---------- Action ----------" {
        # "#CSM \"Category Seperator\"\nDo not put any code in this frame."
        n314 = call <vilib>:"Add State(s) to Queue__JKI_lib_State_Machine.vi"("State(s) in (\"\")"=w786) -> ("States Out"=w785:string)  [unwired: 14 in]
      }
      frame "Action: DISABLE" {
        w789 = T3."Disabled and Grayed Out" ("Disabled")
        # "#CSM \"Internal State\"\nThis category is used for holding internal states"
        n315 = property on="pause" class="Bool (strict)"(error in=w788, "DisabledEnum"=w789) -> (error out=w787:errorcluster)  [unwired: 1 in, 1 out]
        n316 = Unbundle By Name(w798) -> ("Boolean1"=w793:refnum<vi>, "Boolean 3"=w792:refnum<vi>, "Boolean 4"=w791:refnum<vi>, "Boolean 2"=w790:refnum<vi>)
        n317 = property class="Bool (strict)"(reference=w790, error in=w787, "DisabledEnum"=w789) -> (error out=w797:errorcluster)  [unwired: 1 out]
        n318 = property class="Bool (strict)"(reference=w791, error in=w797, "DisabledEnum"=w789) -> (error out=w796:errorcluster)  [unwired: 1 out]
        n319 = property class="Bool (strict)"(reference=w792, error in=w796, "DisabledEnum"=w789) -> (error out=w795:errorcluster)  [unwired: 1 out]
        n320 = property class="Bool (strict)"(reference=w793, error in=w795, "DisabledEnum"=w789) -> (error out=w794:errorcluster)  [unwired: 1 out]
        n321 = call <vilib>:"Add State(s) to Queue__JKI_lib_State_Machine.vi"("State(s) in (\"\")"=w801) -> ("States Out"=w800:string)  [unwired: 14 in]
      }
      frame "Action: ENABLE" {
        w803 = T3."Enabled" ("Disabled")
        # "#CSM \"Internal State\"\nThis category is used for holding internal states"
        n322 = property on="pause" class="Bool (strict)"(error in=w802, "DisabledEnum"=w803) -> (error out=w804:errorcluster)  [unwired: 1 in, 1 out]
        n323 = Unbundle By Name(w810) -> ("Boolean1"=w814:refnum<vi>, "Boolean 3"=w813:refnum<vi>, "Boolean 4"=w812:refnum<vi>, "Boolean 2"=w811:refnum<vi>)
        n324 = property class="Bool (strict)"(reference=w811, error in=w804, "DisabledEnum"=w803) -> (error out=w818:errorcluster)  [unwired: 1 out]
        n325 = property class="Bool (strict)"(reference=w812, error in=w818, "DisabledEnum"=w803) -> (error out=w817:errorcluster)  [unwired: 1 out]
        n326 = property class="Bool (strict)"(reference=w813, error in=w817, "DisabledEnum"=w803) -> (error out=w816:errorcluster)  [unwired: 1 out]
        n327 = Get Date/Time In Seconds() -> (seconds since 1Jan1904=w805:timestamp)
        n328 = property class="Bool (strict)"(reference=w814, error in=w816, "DisabledEnum"=w803) -> (error out=w815:errorcluster)  [unwired: 1 out]
        n329 = call "Convert Data To API String Arguments.vim"("data"=w805) -> ("String"=w807:string)  [unwired: 7 in, 1 out]
        n330 = call-poly <userlib>:"Build Message with Arguments++.vi"("State with Arguments"="API: CNT", "Arguments (\"\")"=w807, "Target Module (\"\")"="Game Engine" ("Target Module (\"\")")) -> ("State with Arguments out"=w809:string)  [unwired: 12 in]
        n331 = call <vilib>:"Add State(s) to Queue__JKI_lib_State_Machine.vi"("State(s) in Front (\"\")"=w809, "State(s) in (\"\")"=w821) -> ("States Out"=w820:string)  [unwired: 13 in]
      }
    }
  }
  n332 = call "User Manage.vi"("Name(\"\" to use uuid)"="User Manage" ("Name(\"\" to use uuid)")) -> ()  [unwired: 11 in]
  n333 = call "Rank.vi"("Name(\"\" to use uuid)"="Rank" ("Name(\"\" to use uuid)")) -> ()  [unwired: 11 in]
  n334 = call "Archive.vi"("Name(\"\" to use uuid)"="Archive" ("Name(\"\" to use uuid)")) -> ()  [unwired: 11 in]
  n335 = call "Game Engine.vi"("Name(\"\" to use uuid)"="Game Engine" ("Name(\"\" to use uuid)")) -> ()  [unwired: 11 in]
